vi "UI_page111.vi"(10 "传递队列输入":refnum<queue>, 11 "notifier":refnum<notifier>) -> ()   [LabVIEW 2012]
uses:
  <vilib>/GPower/VIRegister/Library/Convert/ToSGLArry.vi
  <vilib>/GPower/VIRegister/Library/Convert/ToU32.vi
  <vilib>/GPower/VIRegister/Library/SubVIs/FindRegisterData.vi
  <vilib>/GPower/VIRegister/Library/SubVIs/ReadSub.vi
  <vilib>/GPower/VIRegister/Library/SubVIs/WriteSub.vi
  <vilib>/GPower/VIRegister/Library/QManager/GetRegisterData.vi
  <vilib>/GPower/Error/Library/SetError.vi
  <vilib>/GPower/Error/Library/FilterCodes.vi
  <vilib>/GPower/Error/Library/Filter/FilterMulti.vi
  <vilib>/GPower/VIRegister/Library/QManager/QManagerAction.vi
  <vilib>/GPower/Error/Library/ErrorType.vi
  <vilib>/GPower/Error/Library/SplitAppended.vi
  <vilib>/GPower/Error/Library/SubVIs/ExplanationToError.vi
  <vilib>/GPower/VIRegister/Library/QManager/GetQName.vi
  <vilib>/GPower/VIRegister/Library/QManager/StartQManager.vi
  <vilib>/Utility/error.llb/Trim Whitespace.vi
  <vilib>/dlg_ctls.llb/Space Constant.vi
  <vilib>/Utility/error.llb/Error Code Database.vi
  <vilib>/GPower/Error/Library/SubVIs/SetStatus.vi
  <vilib>/GPower/Error/Library/AppendErrors.vi
  <vilib>/GPower/Error/Library/Append/AppendSingle.vi
  <vilib>/GPower/VIRegister/VIRegister.lvlib
panel:
  in  "备份发送上一指令字":bool
  in  "备份启动自测试":bool
  in  "备份发送自检测试字":bool
  out "备份温控健康状态":bool caption="健康状态"
  out "备份温控工作状态":bool caption="工作状态"
  out "主份温控健康状态":bool caption="健康状态"
  out "主份温控工作状态":bool caption="工作状态"
  in  "主份发送自检测试字":bool
  in  "主份启动自测试":bool
  in  "主份发送上一指令字":bool
  in  "备份地检":bool
  in  "备份1553B":bool=TRUE
  out "备份A3加电状态":bool caption="加电状态"
  out "备份A2加电状态":bool caption="加电状态"
  out "备份A1加电状态":bool caption="加电状态"
  out "备份G3加电状态":bool caption="加电状态"
  out "备份G2加电状态":bool caption="加电状态"
  out "备份G1加电状态":bool caption="加电状态"
  in  "地检":bool
  in  "1553B":bool=TRUE
  out "主份A3加电状态":bool caption="加电状态"
  out "主份A2加电状态":bool caption="加电状态"
  out "主份A1加电状态":bool caption="加电状态"
  out "主份G3加电状态":bool caption="加电状态"
  out "主份G2加电状态":bool caption="加电状态"
  out "主份G1加电状态":bool caption="加电状态"
  in  "主份复位":enum32{"On", "Off"}(radio)=enum."Off" caption="复位"
  in  "备份复位":enum32{"On", "Off"}(radio)=enum."Off" caption="复位"
  in  "备份发送控制字":bool
  in  "主份发送控制字":bool
  in  "备份加计3":enum32{"On", "Off", "Keep"}(radio)=enum."Keep" caption="加计3"
  in  "备份加计2":enum32{"On", "Off", "Keep"}(radio)=enum."Keep" caption="加计2"
  in  "备份加计1":enum32{"On", "Off", "Keep"}(radio)=enum."Keep" caption="加计1"
  in  "备份陀螺3":enum32{"On", "Off", "Keep"}(radio)=enum."Keep" caption="陀螺3"
  in  "备份陀螺2":enum32{"On", "Off", "Keep"}(radio)=enum."Keep" caption="陀螺2"
  in  "备份陀螺1":enum32{"On", "Off", "Keep"}(radio)=enum."Keep" caption="陀螺1"
  in  "备份温控":enum32{"On", "Off", "Keep"}(radio)=enum."Keep" caption="温控"
  in  "加计3":enum32{"On", "Off", "Keep"}(radio)=enum."Keep"
  in  "加计2":enum32{"On", "Off", "Keep"}(radio)=enum."Keep"
  in  "加计1":enum32{"On", "Off", "Keep"}(radio)=enum."Keep"
  in  "陀螺3":enum32{"On", "Off", "Keep"}(radio)=enum."Keep"
  in  "陀螺2":enum32{"On", "Off", "Keep"}(radio)=enum."Keep"
  in  "陀螺1":enum32{"On", "Off", "Keep"}(radio)=enum."Keep"
  in  "温控":enum32{"On", "Off", "Keep"}(radio)=enum."Keep"
  in  "备份切小量程IF电路":bool
  in  "备份切大量程IF电路":bool
  out "模拟量显示区":string
  out "备份自检状态及船舱标志":string
  out "主份自检状态及船舱标志":string
  out "接收数据统计区域":string
  in  "备份复位远程终端":bool
  in  "备份取消发送器关闭":bool
  in  "备份发送器关闭":bool
  in  "备份发送上一状态字":bool
  in  "主份复位远程终端":bool
  in  "主份取消发送器关闭":bool
  in  "主份发送器关闭":bool
  in  "主份发送上一状态字":bool
  in  "备份RT地址选择":enum32{"RT31", "RT21", "RT9"}(radio)
  in  "主份RT地址选择":enum32{"RT31", "RT21", "RT9"}(radio)
  in  "备份通道选择":enum32{"通道A", "通道B"}(radio)
  in  "主份通道选择":enum32{"通道A", "通道B"}(radio)
  in  "备份自定义周期":u16=10 caption="ms" min=10 max=480
  in  "备份周期设置":enum32{"160ms", "自定义", "480ms"}(radio)
  in  "主份自定义周期":u16=10 caption="ms" min=10 max=480
  in  "主份周期设置":enum32{"160ms", "自定义", "480ms"}(radio)
  # "主份模式指令"
  # "备份模式指令"
  # "主份指令"
  # "备份指令"
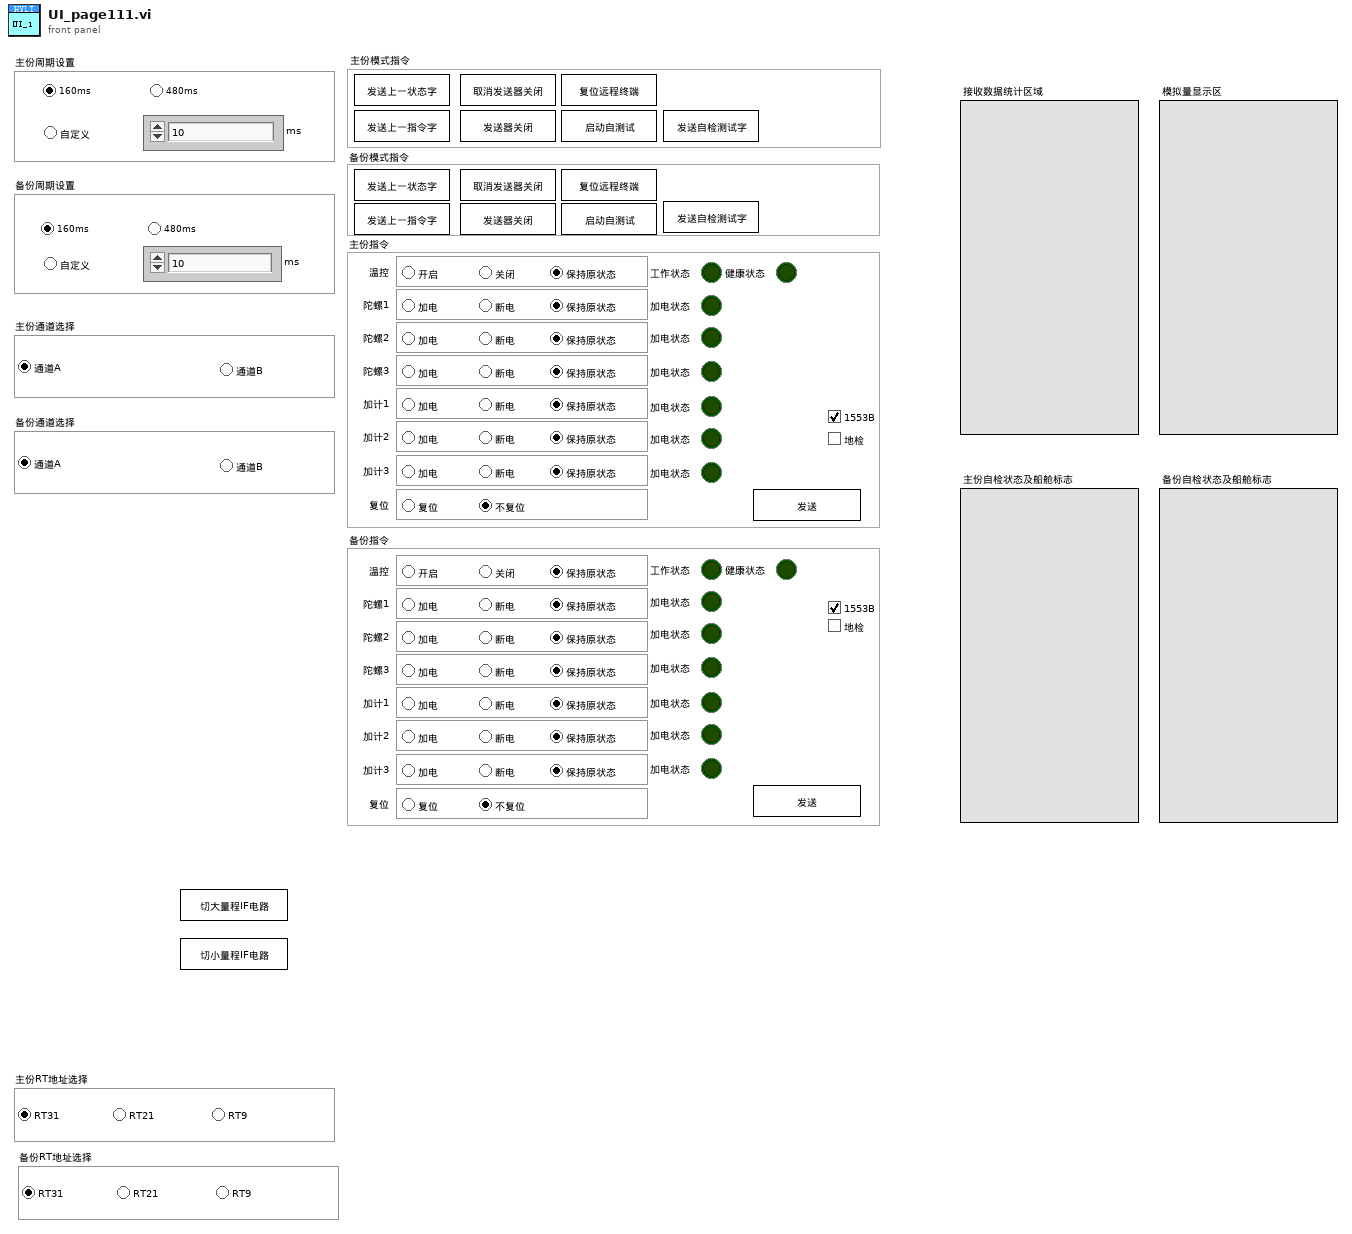
[diagram p1: front panel]
types:
  T1 = cluster{"主份通道选择":enum32{"通道A", "通道B"}, "备份通道选择":enum32{"通道A", "通道B"}}
  T2 = enum32{"invalid app kind", "Development System", "Run Time System", "Student Edition", "Embedded LabVIEW", "Evaluation", "Custom"}
  T3 = enum32{"Invalid", "Standard", "Closed", "Hidden", "Minimized", "Maximized"}
  T4 = cluster{"Core":cluster{"Current VI Reference":refnum<vi>, "Close Panel on Exit?":bool}, "传递队列输入":refnum<queue>, "信息帧":cluster{" 数据帧名称":string, " 数据":string, "备用操作符":bool, "起始地址":i32, "读写标志":i32, "长度":i32}, "主份控制指令":u16, "备份控制指令":u16, "notifier ":refnum<notifier>, "秒计数":i64, "起始时间":i64, "定时控制":bool}
  T5 = cluster{" 数据帧名称":string, " 数据":string, "备用操作符":bool, "起始地址":i32, "读写标志":i32, "长度":i32}
  T6 = cluster{"Current VI Reference":refnum<vi>, "Close Panel on Exit?":bool}
  T7 = cluster{"G1陀螺脉冲数":i32, "G2陀螺脉冲数":i32, "G3陀螺脉冲数":i32, "A1加速度计脉冲数":i16, "A2加速度计脉冲数":i16, "A3加速度计脉冲数":i16, "G1陀螺自检状态":u8, "G1陀螺光路温度":i8, "G2陀螺自检状态":u8, "G2陀螺光路温度":i8, "G3陀螺自检状态":u8, "G3陀螺光路温度":i8, "A1自检状态":u8, "A1幅值":u8, "A2自检状态":u8, "A2幅值":u8, "A3自检状态":u8, "A3幅值":u8, "IF1电路温度":i8, "IF2电路温度":i8, "IF3电路温度":i8, "温控自检字":u8, "加计温度1":i16, "加计温度2":i16, "LTU状态":u8, "帧计数":u8, "G1陀螺光路温度E-2":i16, "G2陀螺光路温度E-2":i16, "G3陀螺光路温度E-2":i16, "G1陀螺电路温度E-2":i16, "G2陀螺电路温度E-2":i16, "G3陀螺电路温度E-2":i16}
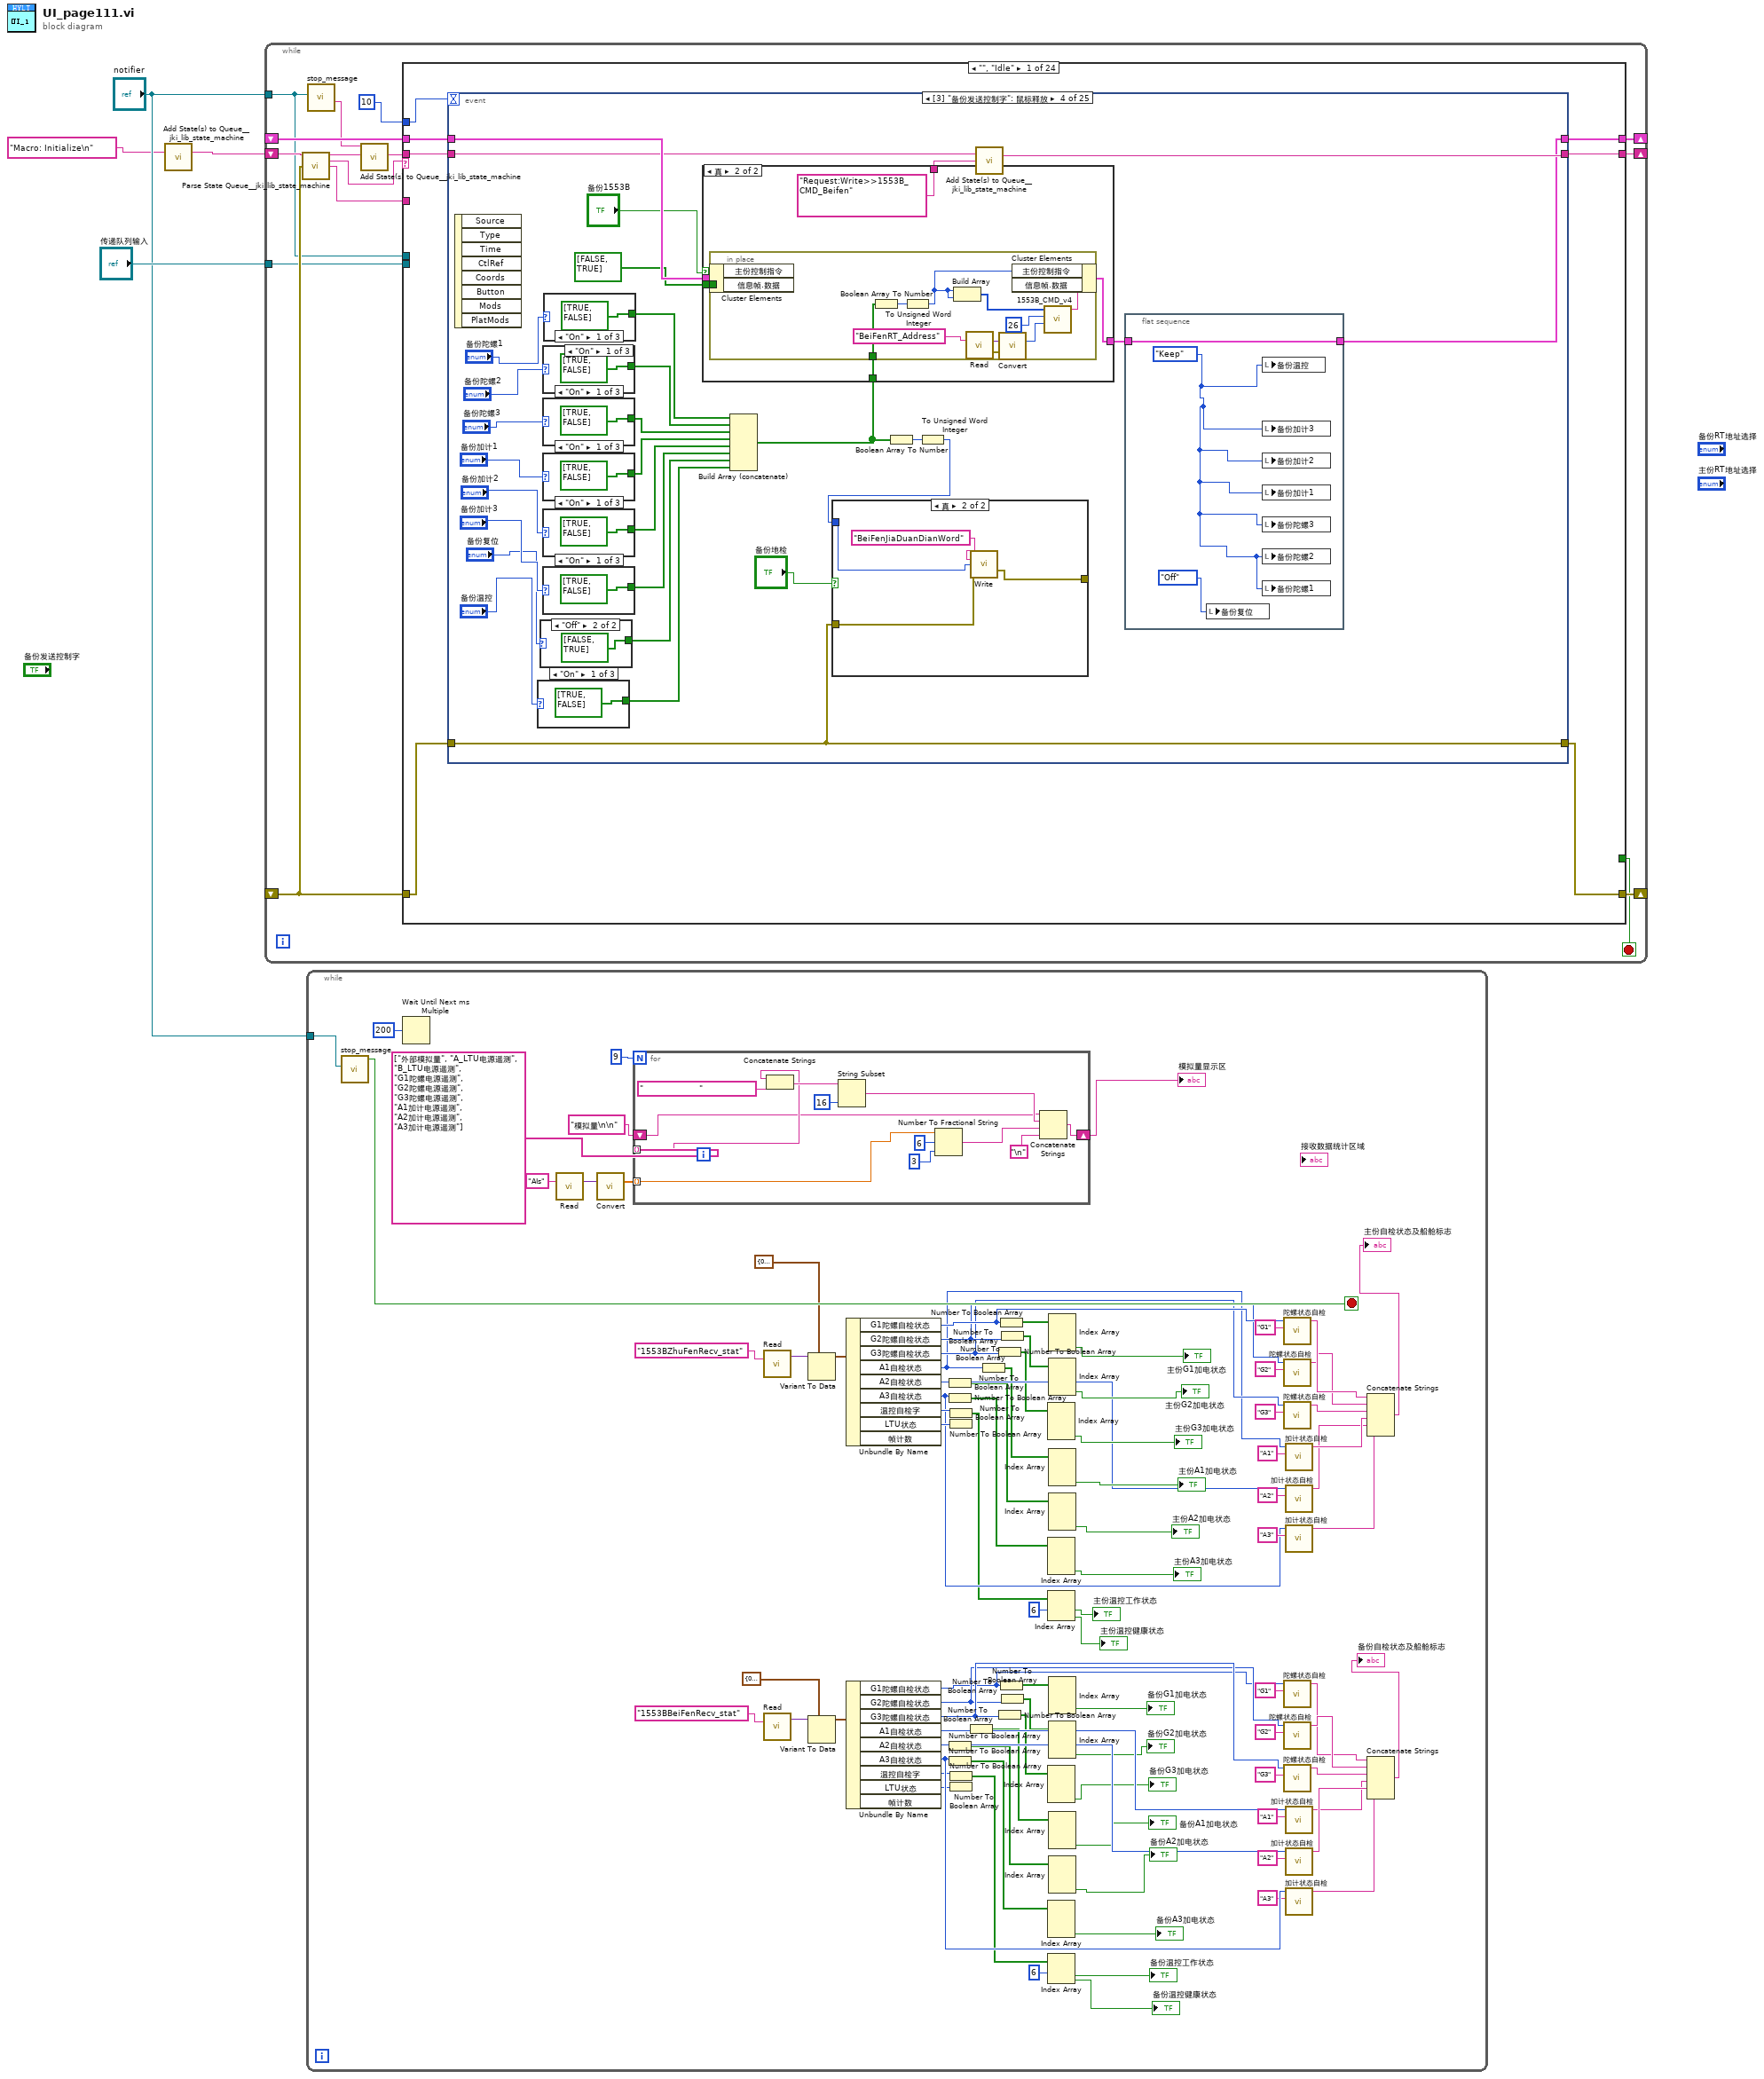
[diagram p0: block diagram]
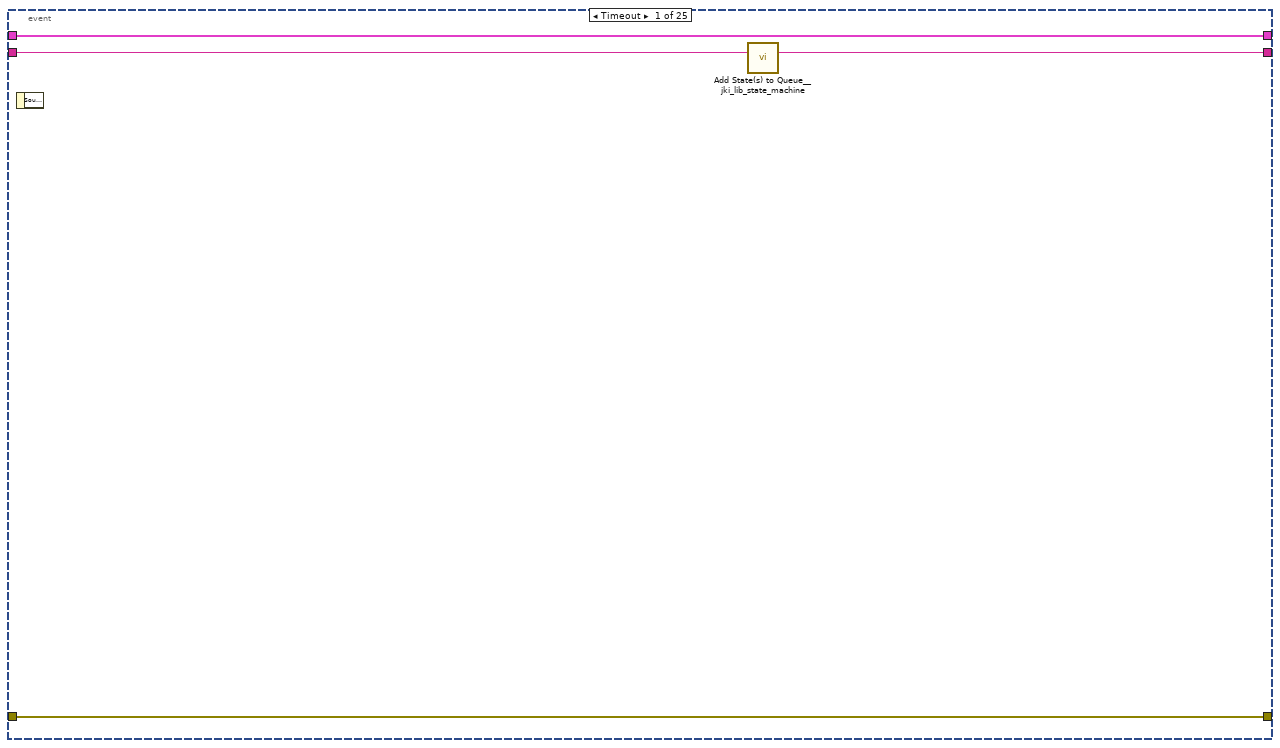
[diagram p2: hidden frame]
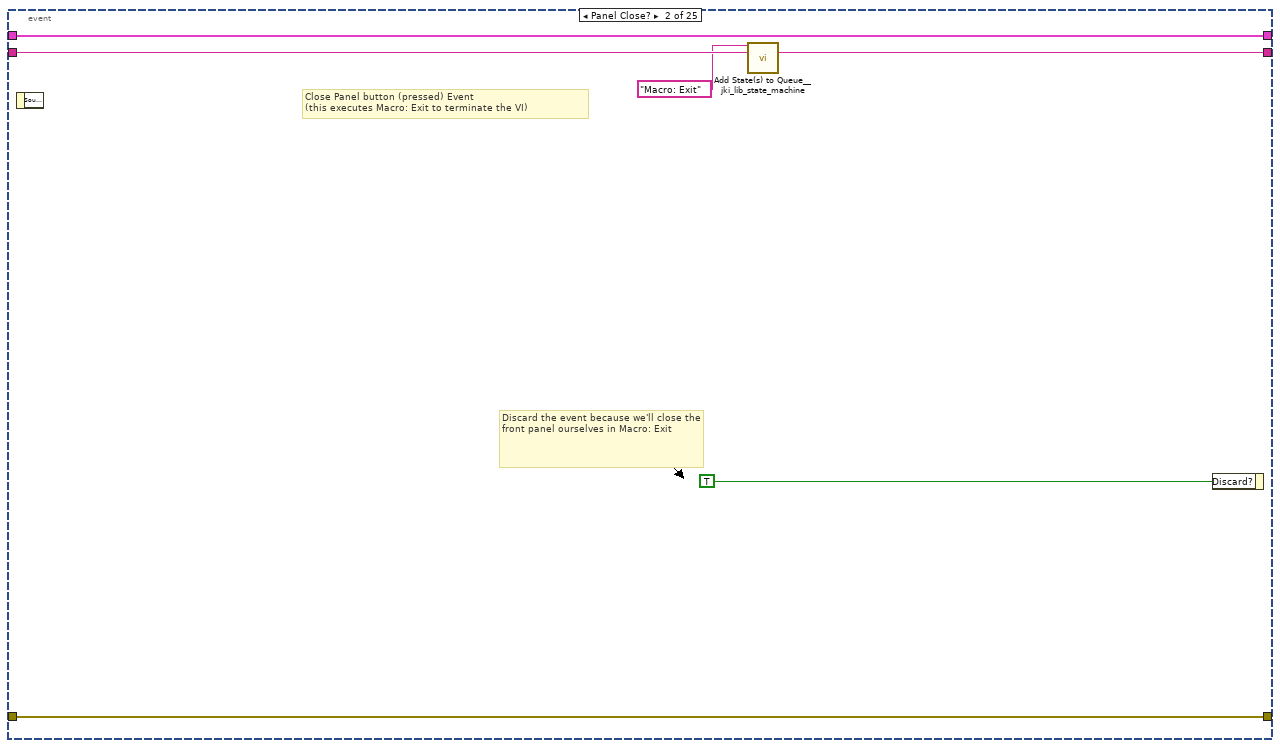
[diagram p3: hidden frame]
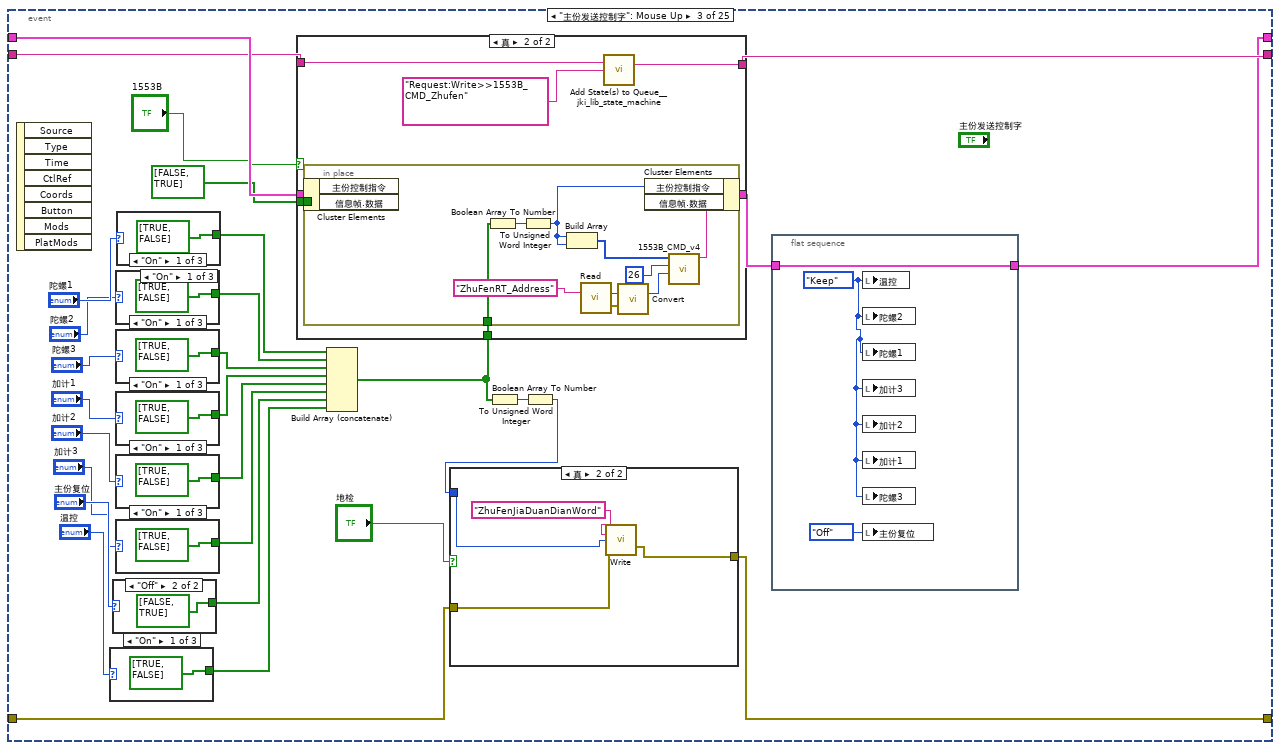
[diagram p4: hidden frame]
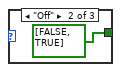
[diagram p7: hidden frame]
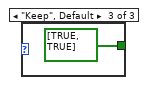
[diagram p8: hidden frame]
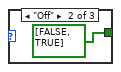
[diagram p9: hidden frame]
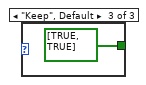
[diagram p10: hidden frame]
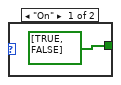
[diagram p11: hidden frame]
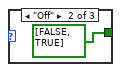
[diagram p12: hidden frame]
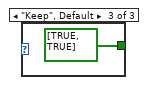
[diagram p13: hidden frame]
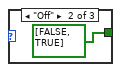
[diagram p14: hidden frame]
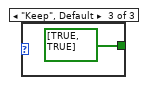
[diagram p15: hidden frame]
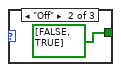
[diagram p16: hidden frame]
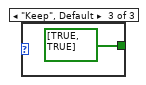
[diagram p17: hidden frame]
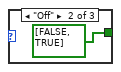
[diagram p18: hidden frame]
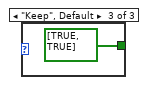
[diagram p19: hidden frame]
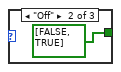
[diagram p20: hidden frame]
diagram:
  n1 = call <vilib>:"Add State(s) to Queue__jki_lib_state_machine.vi"("State(s) in (\"\")"="Macro: Initialize\n") -> ("States Out"=w4:string)  [unwired: 14 in]
  n2 = while "JKI - String-Based Queued State Machine (Basic) v1.0" {
    shift-right: [w13] -> _
    shift-left: _ -> [w12]
    shift-right: [w16] -> _
    shift-left: _ -> [w10]
    shift-right: [w15] -> _
    shift-left: w4 -> [w17]
    tunnel: "notifier" -> [w5]
    tunnel: "传递队列输入" -> [w6]
    stop <- w14 stop-if-true
    n3 = call <vilib>:"Parse State Queue__jki_lib_state_machine.vi"("State Queue"=w17, "Error In (no error)"=w10) -> ("Remaining States"=w9:string, "Current State"=w19:string, "Arguments"=w18:string)  [unwired: 11 in]
    n4 = call "stop_message.vi"("notifier"=w5) -> ("通知"=w8:string)  [unwired: 9 in, 1 out]
    n5 = call <vilib>:"Add State(s) to Queue__jki_lib_state_machine.vi"("State(s) in Front (\"\")"=w8, "State(s) in (\"\")"=w9) -> ("States Out"=w7:string)  [unwired: 13 in]
    n6 = case shown="\"\", \"Idle\"" w19 {
      selector: w19 -> [_ _ w464 _ _ _ _ _ _ _ _ _ _ _ _ _ _ _ _ _ _ _ _ _]
      tunnel: w7 -> [w20 w463 w468 w486 w492 w497 w501 w514 w520 w524 w530 w536 w546 w578 w583 w593 w597 w604 w625 w645 w664 w690 w706 w711]
      tunnel: w18 -> [_ _ _ _ _ _ _ _ _ _ _ w531 w541 _ _ _ _ w598 w619 w639 _ _ _ _]
      tunnel: w12 -> [w25 w460 w466 w477 w489 w495 w498 _ w515 w521 w528 w534 w542 w575 w580 w590 w594 w602 w623 w643 w662 w688 w703 w708]
      tunnel: [w24 w461 w470 w483 errorcluster {"status"=FALSE, "code"=0, "source"=""} ("error out") w494 w499 w511 w516 w522 w527 w532 w543 w576 w581 w591 w595 w600 w621 w641 w660 w686 w704 w709] -> w16
      tunnel: w10 -> [w23 w461 w469 w483 w488 w494 w499 w511 w517 w522 w527 w533 w544 w576 w581 w591 w595 w601 w622 w642 w661 w687 w704 w709]
      tunnel: [w26 w462 w467 w485 w491 w496 w500 w513 w519 w523 w529 w535 w545 w577 w582 w592 w596 w603 w624 w644 w663 w689 w705 w710] -> w15
      tunnel: [_ _ _ _ _ TRUE _ _ _ _ _ _ _ _ _ _ _ _ _ _ _ _ _ _] -> w14
      tunnel: [w22 w460 w466 w484 w489 w495 w498 w512 w515 w521 w528 w534 w542 w575 w580 w590 w594 w599 w620 w640 w659 w685 w703 w708] -> w13
      tunnel: 10 ("Timeout") -> [w21 _ _ _ _ _ _ _ _ _ _ _ _ _ _ _ _ _ _ _ _ _ _ _]
      tunnel: w6 -> [_ _ _ _ _ _ _ w508 _ _ _ _ _ _ _ _ _ _ _ _ _ _ _ _]
      tunnel: w5 -> [_ _ _ _ _ _ _ w505 _ _ _ _ _ _ _ _ _ _ _ _ _ _ _ _]
      frame "", "Idle" {
        n7 = event shown="[3] \"备份发送控制字\": 鼠标释放" {
          selector: _ -> [_ _ _ _ _ _ _ _ _ _ _ _ _ _ _ _ _ _ _ _ _ _ _ _ _]
          dyn-events: _ -> [_ _ _ _ _ _ _ _ _ _ _ _ _ _ _ _ _ _ _ _ _ _ _ _ _]
          timeout: w21 -> [_ _ _ _ _ _ _ _ _ _ _ _ _ _ _ _ _ _ _ _ _ _ _ _ _]
          tunnel: w20 -> [w30 w36 w64 w143 w199 w208 w215 w236 w255 w273 w284 w295 w307 w319 w331 w343 w355 w367 w379 w391 w403 w415 w427 w439 w451]
          tunnel: [w29 w35 w63 w141 w197 w206 w214 w235 w254 w272 w282 w293 w305 w317 w329 w341 w353 w365 w377 w389 w401 w413 w425 w437 w449] -> w26
          tunnel: w25 -> [w27 w33 w65 w144 w201 w210 w218 w238 w257 w270 w286 w297 w309 w321 w333 w345 w357 w369 w381 w393 w405 w417 w429 w441 w453]
          tunnel: [w28 w34 w37 w117 w196 w205 w213 w227 w246 w265 w281 w292 w304 w316 w328 w340 w352 w364 w376 w388 w400 w412 w424 w436 w448] -> w24
          tunnel: w23 -> [w28 w34 w38 w117 w196 w205 w213 w231 w249 w266 w281 w292 w304 w316 w328 w340 w352 w364 w376 w388 w400 w412 w424 w436 w448]
          tunnel: [w27 w33 w44 w130 w200 w209 w216 w237 w256 w269 w285 w296 w308 w320 w332 w344 w356 w368 w380 w392 w404 w416 w428 w440 w452] -> w22
          event Timeout {
            n8 = event-data() -> ()  [unwired: 1 in, 1 out]
            n9 = call <vilib>:"Add State(s) to Queue__jki_lib_state_machine.vi"("State(s) in (\"\")"=w30) -> ("States Out"=w29:string)  [unwired: 14 in]
          }
          event Panel Close? {
            # "Discard the event because we'll close the front panel ourselves in Macro: Exit"
            # "Close Panel button (pressed) Event\n(this executes Macro: Exit to terminate the VI)"
            n10 = event-data() -> ()  [unwired: 1 in, 1 out]
            n11 = call <vilib>:"Add State(s) to Queue__jki_lib_state_machine.vi"("State(s) in Front (\"\")"="Macro: Exit", "State(s) in (\"\")"=w36) -> ("States Out"=w35:string)  [unwired: 13 in]
            n12 = event-data("Discard?"=TRUE) -> ()  [unwired: 1 in, 1 out]
          }
          event "主份发送控制字": Mouse Up {
            n13 = event-data() -> ()  [unwired: 1 in, 8 out]
            n14 = case shown="\"On\"" "温控" {
              tunnel: [bool[] [TRUE, FALSE] bool[] [FALSE, TRUE] bool[] [TRUE, TRUE]] -> w46
              frame "On" {
              }
              frame "Off" {
              }
              frame "Keep", Default {
              }
            }
            n15 = case shown="\"Off\"" "主份复位" {
              tunnel: [bool[] [TRUE, FALSE] bool[] [FALSE, TRUE]] -> w47
              frame "On" {
              }
              frame "Off" {
              }
            }
            n16 = case shown="\"On\"" "陀螺2" {
              tunnel: [bool[] [TRUE, FALSE] bool[] [FALSE, TRUE] bool[] [TRUE, TRUE]] -> w52
              frame "On" {
              }
              frame "Off" {
              }
              frame "Keep", Default {
              }
            }
            n17 = case shown="\"On\"" "陀螺3" {
              tunnel: [bool[] [TRUE, FALSE] bool[] [FALSE, TRUE] bool[] [TRUE, TRUE]] -> w51
              frame "On" {
              }
              frame "Off" {
              }
              frame "Keep", Default {
              }
            }
            n18 = case shown="\"On\"" "加计1" {
              tunnel: [bool[] [TRUE, FALSE] bool[] [FALSE, TRUE] bool[] [TRUE, TRUE]] -> w50
              frame "On" {
              }
              frame "Off" {
              }
              frame "Keep", Default {
              }
            }
            n19 = case shown="\"On\"" "加计2" {
              tunnel: [bool[] [TRUE, FALSE] bool[] [FALSE, TRUE] bool[] [TRUE, TRUE]] -> w49
              frame "On" {
              }
              frame "Off" {
              }
              frame "Keep", Default {
              }
            }
            n20 = case shown="\"On\"" "加计3" {
              tunnel: [bool[] [TRUE, FALSE] bool[] [FALSE, TRUE] bool[] [TRUE, TRUE]] -> w48
              frame "On" {
              }
              frame "Off" {
              }
              frame "Keep", Default {
              }
            }
            n21 = case shown="\"On\"" "陀螺1" {
              tunnel: [bool[] [TRUE, FALSE] bool[] [FALSE, TRUE] bool[] [TRUE, TRUE]] -> w53
              frame "On" {
              }
              frame "Off" {
              }
              frame "Keep", Default {
              }
            }
            n22 = Build Array (concatenate)(w53, w52, w51, w50, w49, w48, w47, w46) -> (w41:bool[])
            n23 = case shown="真" "1553B" {
              tunnel: w65 -> [w71 w79]
              tunnel: w64 -> [w72 w78]
              tunnel: [w72 w76] -> w63
              tunnel: bool[] [FALSE, TRUE] -> [_ w75]
              tunnel: w41 -> [_ w74]
              tunnel: [w71 w73] -> w45
              frame False {
              }
              frame True {
                n24 = in-place {
                  in-place-border: w75 -> [_]
                  in-place-border: w74 -> [w88]
                  n25 = in-place-cluster #1(w79) -> ()  [unwired: 2 out]
                  n26 = Boolean Array To Number(Boolean array=w88) -> (number=w89:u32)
                  n27 = To Unsigned Word Integer(number=w89) -> (unsigned 16bit integer=w80:u16)
                  n28 = Build Array(w80, w80) -> (w86:u16[])
                  n29 = call <vilib>:"Read.vi"("Register name"="ZhuFenRT_Address") -> ("Register value"=w84:variant, "Error out"=w81:errorcluster)  [unwired: 11 in, 2 out]
                  n30 = call-poly <vilib>:"Convert.vi"("Register value in"=w84, "Error in"=w81) -> ("Register value out"=w83:u32)  [unwired: 12 in, 1 out]
                  n31 = call "1553B_CMD_v4.vi"("RT地址"=w83, "控制指令子地址(默认：11010"=u16 26, "数据字数组"=w86) -> ("1553B指令"=w82:string)  [unwired: 8 in]
                  n32 = in-place-cluster #1("主份控制指令"=w80, "信息帧.数据"=w82) -> (w73:T4)
                }
                n33 = call <vilib>:"Add State(s) to Queue__jki_lib_state_machine.vi"("State(s) in (\"\")"=w78, "State(s) at Back (\"\")"="Request:Write>>1553B_CMD_Zhufen") -> ("States Out"=w76:string)  [unwired: 13 in]
              }
            }
            n34 = Boolean Array To Number(Boolean array=w41) -> (number=w42:u32)
            n35 = To Unsigned Word Integer(number=w42) -> (unsigned 16bit integer=w39:u16)
            n36 = case shown="真" "地检" {
              tunnel: w39 -> [_ w69]
              tunnel: w38 -> [w66 w68]
              tunnel: [w66 w67] -> w37
              frame False {
              }
              frame True {
                n37 = call <vilib>:"Write.vi"("Register name"="ZhuFenJiaDuanDianWord", "Register value"=w69, "Error in"=w68) -> ("Error out"=w67:errorcluster)  [unwired: 10 in, 2 out]
              }
            }
            n38 = flat-sequence {
              tunnel: w45 -> [w90]
              tunnel: [w90] -> w44
              frame #0 {
                w92 = enum32{"On", "Off", "Keep"}."Keep" ("温控")
                n39 = local write "温控"(w92) -> ()
                n40 = local write "陀螺2"(w92) -> ()
                n41 = local write "陀螺1"(w92) -> ()
                n42 = local write "加计3"(w92) -> ()
                n43 = local write "加计2"(w92) -> ()
                n44 = local write "加计1"(w92) -> ()
                n45 = local write "陀螺3"(w92) -> ()
                n46 = local write "主份复位"(enum32{"On", "Off"}."Off" ("主份复位")) -> ()
              }
            }
          }
          event "备份发送控制字": Mouse Up {
            n47 = event-data() -> ()  [unwired: 1 in, 8 out]
            n48 = case shown="\"On\"" "备份温控" {
              tunnel: [bool[] [TRUE, FALSE] bool[] [FALSE, TRUE] bool[] [TRUE, TRUE]] -> w132
              frame "On" {
              }
              frame "Off" {
              }
              frame "Keep", Default {
              }
            }
            n49 = case shown="\"Off\"" "备份复位" {
              tunnel: [bool[] [TRUE, FALSE] bool[] [FALSE, TRUE]] -> w133
              frame "On" {
              }
              frame "Off" {
              }
            }
            n50 = case shown="\"On\"" "备份陀螺2" {
              tunnel: [bool[] [TRUE, FALSE] bool[] [FALSE, TRUE] bool[] [TRUE, TRUE]] -> w138
              frame "On" {
              }
              frame "Off" {
              }
              frame "Keep", Default {
              }
            }
            n51 = case shown="\"On\"" "备份陀螺3" {
              tunnel: [bool[] [TRUE, FALSE] bool[] [FALSE, TRUE] bool[] [TRUE, TRUE]] -> w137
              frame "On" {
              }
              frame "Off" {
              }
              frame "Keep", Default {
              }
            }
            n52 = case shown="\"On\"" "备份加计1" {
              tunnel: [bool[] [TRUE, FALSE] bool[] [FALSE, TRUE] bool[] [TRUE, TRUE]] -> w136
              frame "On" {
              }
              frame "Off" {
              }
              frame "Keep", Default {
              }
            }
            n53 = case shown="\"On\"" "备份加计2" {
              tunnel: [bool[] [TRUE, FALSE] bool[] [FALSE, TRUE] bool[] [TRUE, TRUE]] -> w135
              frame "On" {
              }
              frame "Off" {
              }
              frame "Keep", Default {
              }
            }
            n54 = case shown="\"On\"" "备份加计3" {
              tunnel: [bool[] [TRUE, FALSE] bool[] [FALSE, TRUE] bool[] [TRUE, TRUE]] -> w134
              frame "On" {
              }
              frame "Off" {
              }
              frame "Keep", Default {
              }
            }
            n55 = case shown="\"On\"" "备份陀螺1" {
              tunnel: [bool[] [TRUE, FALSE] bool[] [FALSE, TRUE] bool[] [TRUE, TRUE]] -> w139
              frame "On" {
              }
              frame "Off" {
              }
              frame "Keep", Default {
              }
            }
            n56 = Build Array (concatenate)(w139, w138, w137, w136, w135, w134, w133, w132) -> (w119:bool[])
            n57 = case shown="真" "备份1553B" {
              tunnel: w144 -> [w145 w151]
              tunnel: ["" "Request:Write>>1553B_CMD_Beifen"] -> w142
              tunnel: bool[] [FALSE, TRUE] -> [_ w149]
              tunnel: [w145 w148] -> w131
              tunnel: w119 -> [_ w147]
              frame False {
              }
              frame True {
                n58 = in-place {
                  in-place-border: w149 -> [_]
                  in-place-border: w147 -> [w160]
                  n59 = in-place-cluster #2(w151) -> ()  [unwired: 2 out]
                  n60 = Boolean Array To Number(Boolean array=w160) -> (number=w161:u32)
                  n61 = To Unsigned Word Integer(number=w161) -> (unsigned 16bit integer=w152:u16)
                  n62 = Build Array(w152, w152) -> (w158:u16[])
                  n63 = call <vilib>:"Read.vi"("Register name"="BeiFenRT_Address") -> ("Register value"=w157:variant, "Error out"=w155:errorcluster)  [unwired: 11 in, 2 out]
                  n64 = call-poly <vilib>:"Convert.vi"("Register value in"=w157, "Error in"=w155) -> ("Register value out"=w156:u32)  [unwired: 12 in, 1 out]
                  n65 = call "1553B_CMD_v4.vi"("RT地址"=w156, "控制指令子地址(默认：11010"=u16 26, "数据字数组"=w158) -> ("1553B指令"=w153:string)  [unwired: 8 in]
                  n66 = in-place-cluster #2("主份控制指令"=w152, "信息帧.数据"=w153) -> (w148:T4)
                }
              }
            }
            n67 = Boolean Array To Number(Boolean array=w119) -> (number=w120:u32)
            n68 = To Unsigned Word Integer(number=w120) -> (unsigned 16bit integer=w118:u16)
            n69 = case shown="真" "备份地检" {
              tunnel: w118 -> [_ w165]
              tunnel: w117 -> [w162 w164]
              tunnel: [w162 w163] -> _
              frame False {
              }
              frame True {
                n70 = call <vilib>:"Write.vi"("Register name"="BeiFenJiaDuanDianWord", "Register value"=w165, "Error in"=w164) -> ("Error out"=w163:errorcluster)  [unwired: 10 in, 2 out]
              }
            }
            n71 = call <vilib>:"Add State(s) to Queue__jki_lib_state_machine.vi"("State(s) in (\"\")"=w143, "State(s) at Back (\"\")"=w142) -> ("States Out"=w141:string)  [unwired: 13 in]
            n72 = flat-sequence {
              tunnel: w131 -> [w169]
              tunnel: [w169] -> w130
              frame #0 {
                w167 = enum32{"On", "Off", "Keep"}."Keep" ("温控")
                n73 = local write "备份复位"(enum32{"On", "Off"}."Off" ("主份复位")) -> ()
                n74 = local write "备份温控"(w167) -> ()
                n75 = local write "备份加计3"(w167) -> ()
                n76 = local write "备份加计2"(w167) -> ()
                n77 = local write "备份加计1"(w167) -> ()
                n78 = local write "备份陀螺3"(w167) -> ()
                n79 = local write "备份陀螺2"(w167) -> ()
                n80 = local write "备份陀螺1"(w167) -> ()
              }
            }
          }
          event "备份切大量程IF电路": Value Change {
            n81 = event-data() -> ()  [unwired: 1 in, 6 out]
            n82 = call "1553B_CMD_v4.vi"("控制指令子地址(默认：11010"=u16 26, "数据字数组"=u16[] [45489]) -> ("1553B指令"=w193:string)  [unwired: 9 in]
            n83 = call <vilib>:"Add State(s) to Queue__jki_lib_state_machine.vi"("State(s) in (\"\")"=w199, "State(s) at Back (\"\")"="Request:Write>>1553B_CMD_Beifen") -> ("States Out"=w197:string)  [unwired: 13 in]
            n84 = Bundle By Name(cluster=w201, "信息帧.数据"=w193) -> (w200:T4)
          }
          event "备份切小量程IF电路": Value Change {
            n85 = event-data() -> ()  [unwired: 1 in, 6 out]
            n86 = call "1553B_CMD_v4.vi"("控制指令子地址(默认：11010"=u16 26, "数据字数组"=u16[] [47802]) -> ("1553B指令"=w202:string)  [unwired: 9 in]
            n87 = call <vilib>:"Add State(s) to Queue__jki_lib_state_machine.vi"("State(s) in (\"\")"=w208, "State(s) at Back (\"\")"="Request:Write>>1553B_CMD_Beifen") -> ("States Out"=w206:string)  [unwired: 13 in]
            n88 = Bundle By Name(cluster=w210, "信息帧.数据"=w202) -> (w209:T4)
          }
          event "主份自定义周期": Value Change {
            n89 = event-data() -> ("NewVal"=w217:u16)  [unwired: 1 in, 5 out]
            n90 = property on="主份周期设置" class="RadioBtnsControl (严格)"() -> ("Value"=w212:enum32{"160ms", "自定义", "480ms"})  [unwired: 2 in, 2 out]
            n91 = case shown="\"自定义\"" w212 {
              tunnel: w218 -> [w220 w226]
              tunnel: w217 -> [_ w221]
              tunnel: [w220 w225] -> w216
              tunnel: ["" "Config:Write>>1553B_CMD_Zhufen"] -> w211
              frame "160ms", Default {
              }
              frame "自定义" {
                n92 = Number To Decimal String(number=w221) -> (decimal integer string=w224:string)  [unwired: 1 in]
                n93 = Bundle By Name(cluster=w226, "信息帧.数据"=w224) -> (w225:T4)
                n94 = call <vilib>:"Write.vi"("Register name"="Zhufen_period", "Register value"=w221) -> ()  [unwired: 11 in, 3 out]
              }
            }
            n95 = call <vilib>:"Add State(s) to Queue__jki_lib_state_machine.vi"("State(s) in (\"\")"=w215, "State(s) at Back (\"\")"=w211) -> ("States Out"=w214:string)  [unwired: 13 in]
          }
          event "主份周期设置": Value Change {
            n96 = event-data() -> ("NewVal"=w233:enum32{"160ms", "自定义", "480ms"})  [unwired: 1 in, 5 out]
            n97 = case shown="\"自定义\"" w233 {
              tunnel: [u16 160 ("Value") u16 480 ("Value") w245] -> w229
              tunnel: w231 -> [w239 w241 w244]
              tunnel: [w239 w241 w243] -> w228
              frame "160ms", Default {
              }
              frame "480ms" {
              }
              frame "自定义" {
                n98 = property on="主份自定义周期" class="DigNum (严格)"(error in=w244) -> (error out=w243:errorcluster, "Value"=w245:u16)  [unwired: 1 in, 1 out]
              }
            }
            n99 = Number To Decimal String(number=w229) -> (decimal integer string=w232:string)  [unwired: 1 in]
            n100 = Bundle By Name(cluster=w238, "信息帧.数据"=w232) -> (w237:T4)
            n101 = call <vilib>:"Add State(s) to Queue__jki_lib_state_machine.vi"("State(s) in (\"\")"=w236, "State(s) at Back (\"\")"="Config:Write>>1553B_CMD_Zhufen") -> ("States Out"=w235:string)  [unwired: 13 in]
            n102 = call <vilib>:"Write.vi"("Register name"="Zhufen_period", "Register value"=w229, "Error in"=w228) -> ("Error out"=w227:errorcluster)  [unwired: 10 in, 2 out]
          }
          event "备份周期设置": Value Change {
            n103 = event-data() -> ("NewVal"=w248:enum32{"160ms", "自定义", "480ms"})  [unwired: 1 in, 5 out]
            n104 = case shown="\"480ms\"" w248 {
              tunnel: [u16 160 ("Value") u16 480 ("Value") w264] -> w251
              tunnel: w249 -> [w258 w260 w263]
              tunnel: [w258 w260 w262] -> w250
              frame "160ms", Default {
              }
              frame "480ms" {
              }
              frame "自定义" {
                n105 = property on="备份自定义周期" class="DigNum (严格)"(error in=w263) -> (error out=w262:errorcluster, "Value"=w264:u16)  [unwired: 1 in, 1 out]
              }
            }
            n106 = call <vilib>:"Add State(s) to Queue__jki_lib_state_machine.vi"("State(s) in (\"\")"=w255, "State(s) at Back (\"\")"="Config:Write>>1553B_CMD_Beifen") -> ("States Out"=w254:string)  [unwired: 13 in]
            n107 = Number To Decimal String(number=w251) -> (decimal integer string=w247:string)  [unwired: 1 in]
            n108 = Bundle By Name(cluster=w257, "信息帧.数据"=w247) -> (w256:T4)
            n109 = call <vilib>:"Write.vi"("Register name"="Beifen_period", "Register value"=w251, "Error in"=w250) -> ("Error out"=w246:errorcluster)  [unwired: 10 in, 2 out]
          }
          event "备份自定义周期": Value Change {
            n110 = event-data() -> ("NewVal"=w268:u16)  [unwired: 1 in, 5 out]
            n111 = property on="备份周期设置" class="RadioBtnsControl (严格)"(error in=w266) -> (error out=w265:errorcluster, "Value"=w267:enum32{"160ms", "自定义", "480ms"})  [unwired: 1 in, 1 out]
            n112 = case shown="\"自定义\"" w267 {
              tunnel: w270 -> [w275 w280]
              tunnel: w268 -> [_ w279]
              tunnel: [w275 w278] -> w269
              tunnel: ["" "Config:Write>>1553B_CMD_Beifen"] -> w271
              frame "160ms", Default {
              }
              frame "自定义" {
                n113 = Number To Decimal String(number=w279) -> (decimal integer string=w277:string)  [unwired: 1 in]
                n114 = Bundle By Name(cluster=w280, "信息帧.数据"=w277) -> (w278:T4)
              }
            }
            n115 = call <vilib>:"Add State(s) to Queue__jki_lib_state_machine.vi"("State(s) in (\"\")"=w273, "State(s) at Back (\"\")"=w271) -> ("States Out"=w272:string)  [unwired: 13 in]
          }
          event "主份通道选择", "备份通道选择": Value Change {
            # "Request:OPEN1553B>>1553B_CMD_Zhufen\nRequest:OPEN1553B>>1553B_CMD_Beifen"
            n116 = event-data() -> ()  [unwired: 1 in, 6 out]
            n117 = in-place {
              n118 = in-place-cluster #3(w286) -> ()  [unwired: 1 out]
              n119 = Bundle By Name(cluster=T1 {"主份通道选择"=enum."通道A", "备份通道选择"=enum."通道B"} ("输入簇"), "主份通道选择"="主份通道选择", "备份通道选择"="备份通道选择") -> (w288:T1)
              n120 = Flatten To String(anything=w288) -> (data string=w287:string)  [unwired: 3 in, 2 out]
              n121 = in-place-cluster #3("信息帧.数据"=w287) -> (w285:T4)
            }
            n122 = call <vilib>:"Add State(s) to Queue__jki_lib_state_machine.vi"("State(s) in (\"\")"=w284, "State(s) at Back (\"\")"="Request:Write>>SwitchChanel\n") -> ("States Out"=w282:string)  [unwired: 13 in]
          }
          event "主份复位远程终端": Value Change {
            n123 = event-data() -> ()  [unwired: 1 in, 6 out]
            n124 = in-place {
              n125 = in-place-cluster #4(w297) -> ()  [unwired: 1 out]
              n126 = call <vilib>:"Read.vi"("Register name"="ZhuFenRT_Address") -> ("Register value"=w301:variant, "Error out"=w300:errorcluster)  [unwired: 11 in, 2 out]
              n127 = call-poly <vilib>:"Convert.vi"("Register value in"=w301, "Error in"=w300) -> ("Register value out"=w298:u32)  [unwired: 12 in, 1 out]
              n128 = call "1553B_Mode.vi"("模式命令"=u16 8, "RT地址"=w298) -> ("1553B指令"=w302:string)  [unwired: 9 in]
              n129 = in-place-cluster #4("信息帧.数据"=w302) -> (w296:T4)
            }
            n130 = call <vilib>:"Add State(s) to Queue__jki_lib_state_machine.vi"("State(s) in (\"\")"=w295, "State(s) at Back (\"\")"="Request:Write>>1553B_CMD_Zhufen") -> ("States Out"=w293:string)  [unwired: 13 in]
          }
          event "备份复位远程终端": Value Change {
            n131 = event-data() -> ()  [unwired: 1 in, 6 out]
            n132 = in-place {
              n133 = in-place-cluster #5(w309) -> ()  [unwired: 1 out]
              n134 = call <vilib>:"Read.vi"("Register name"="BeiFenRT_Address") -> ("Register value"=w314:variant, "Error out"=w313:errorcluster)  [unwired: 11 in, 2 out]
              n135 = call-poly <vilib>:"Convert.vi"("Register value in"=w314, "Error in"=w313) -> ("Register value out"=w312:u32)  [unwired: 12 in, 1 out]
              n136 = call "1553B_Mode.vi"("模式命令"=u16 8, "RT地址"=w312) -> ("1553B指令"=w311:string)  [unwired: 9 in]
              n137 = in-place-cluster #5("信息帧.数据"=w311) -> (w308:T4)
            }
            n138 = call <vilib>:"Add State(s) to Queue__jki_lib_state_machine.vi"("State(s) in (\"\")"=w307, "State(s) at Back (\"\")"="Request:Write>>1553B_CMD_Beifen") -> ("States Out"=w305:string)  [unwired: 13 in]
          }
          event "主份发送器关闭": Value Change {
            n139 = event-data() -> ()  [unwired: 1 in, 6 out]
            n140 = in-place {
              n141 = in-place-cluster #6(w321) -> ()  [unwired: 1 out]
              n142 = call <vilib>:"Read.vi"("Register name"="ZhuFenRT_Address") -> ("Register value"=w325:variant, "Error out"=w324:errorcluster)  [unwired: 11 in, 2 out]
              n143 = call-poly <vilib>:"Convert.vi"("Register value in"=w325, "Error in"=w324) -> ("Register value out"=w322:u32)  [unwired: 12 in, 1 out]
              n144 = call "1553B_Mode.vi"("模式命令"=u16 4, "RT地址"=w322) -> ("1553B指令"=w326:string)  [unwired: 9 in]
              n145 = in-place-cluster #6("信息帧.数据"=w326) -> (w320:T4)
            }
            n146 = call <vilib>:"Add State(s) to Queue__jki_lib_state_machine.vi"("State(s) in (\"\")"=w319, "State(s) at Back (\"\")"="Request:Write>>1553B_CMD_Zhufen") -> ("States Out"=w317:string)  [unwired: 13 in]
          }
          event "主份发送上一指令字": Value Change {
            n147 = event-data() -> ()  [unwired: 1 in, 6 out]
            n148 = in-place {
              n149 = in-place-cluster #7(w333) -> ()  [unwired: 1 out]
              n150 = call <vilib>:"Read.vi"("Register name"="ZhuFenRT_Address") -> ("Register value"=w337:variant, "Error out"=w336:errorcluster)  [unwired: 11 in, 2 out]
              n151 = call-poly <vilib>:"Convert.vi"("Register value in"=w337, "Error in"=w336) -> ("Register value out"=w334:u32)  [unwired: 12 in, 1 out]
              n152 = call "1553B_Mode.vi"("模式命令"=u16 18, "RT地址"=w334) -> ("1553B指令"=w338:string)  [unwired: 9 in]
              n153 = in-place-cluster #7("信息帧.数据"=w338) -> (w332:T4)
            }
            n154 = call <vilib>:"Add State(s) to Queue__jki_lib_state_machine.vi"("State(s) in (\"\")"=w331, "State(s) at Back (\"\")"="Request:Write>>1553B_CMD_Zhufen") -> ("States Out"=w329:string)  [unwired: 13 in]
          }
          event "备份发送上一指令字": Value Change {
            n155 = event-data() -> ()  [unwired: 1 in, 6 out]
            n156 = in-place {
              n157 = in-place-cluster #8(w345) -> ()  [unwired: 1 out]
              n158 = call <vilib>:"Read.vi"("Register name"="BeiFenRT_Address") -> ("Register value"=w349:variant, "Error out"=w348:errorcluster)  [unwired: 11 in, 2 out]
              n159 = call-poly <vilib>:"Convert.vi"("Register value in"=w349, "Error in"=w348) -> ("Register value out"=w346:u32)  [unwired: 12 in, 1 out]
              n160 = call "1553B_Mode.vi"("模式命令"=u16 18, "RT地址"=w346) -> ("1553B指令"=w350:string)  [unwired: 9 in]
              n161 = in-place-cluster #8("信息帧.数据"=w350) -> (w344:T4)
            }
            n162 = call <vilib>:"Add State(s) to Queue__jki_lib_state_machine.vi"("State(s) in (\"\")"=w343, "State(s) at Back (\"\")"="Request:Write>>1553B_CMD_Zhufen") -> ("States Out"=w341:string)  [unwired: 13 in]
          }
          event "主份启动自测试": Value Change {
            n163 = event-data() -> ()  [unwired: 1 in, 6 out]
            n164 = in-place {
              n165 = in-place-cluster #9(w357) -> ()  [unwired: 1 out]
              n166 = call <vilib>:"Read.vi"("Register name"="ZhuFenRT_Address") -> ("Register value"=w361:variant, "Error out"=w360:errorcluster)  [unwired: 11 in, 2 out]
              n167 = call-poly <vilib>:"Convert.vi"("Register value in"=w361, "Error in"=w360) -> ("Register value out"=w358:u32)  [unwired: 12 in, 1 out]
              n168 = call "1553B_Mode.vi"("模式命令"=u16 3, "RT地址"=w358) -> ("1553B指令"=w362:string)  [unwired: 9 in]
              n169 = in-place-cluster #9("信息帧.数据"=w362) -> (w356:T4)
            }
            n170 = call <vilib>:"Add State(s) to Queue__jki_lib_state_machine.vi"("State(s) in (\"\")"=w355, "State(s) at Back (\"\")"="Request:Write>>1553B_CMD_Zhufen") -> ("States Out"=w353:string)  [unwired: 13 in]
          }
          event "备份启动自测试": Value Change {
            n171 = event-data() -> ()  [unwired: 1 in, 6 out]
            n172 = in-place {
              n173 = in-place-cluster #10(w369) -> ()  [unwired: 1 out]
              n174 = call <vilib>:"Read.vi"("Register name"="BeiFenRT_Address") -> ("Register value"=w373:variant, "Error out"=w372:errorcluster)  [unwired: 11 in, 2 out]
              n175 = call-poly <vilib>:"Convert.vi"("Register value in"=w373, "Error in"=w372) -> ("Register value out"=w370:u32)  [unwired: 12 in, 1 out]
              n176 = call "1553B_Mode.vi"("模式命令"=u16 3, "RT地址"=w370) -> ("1553B指令"=w374:string)  [unwired: 9 in]
              n177 = in-place-cluster #10("信息帧.数据"=w374) -> (w368:T4)
            }
            n178 = call <vilib>:"Add State(s) to Queue__jki_lib_state_machine.vi"("State(s) in (\"\")"=w367, "State(s) at Back (\"\")"="Request:Write>>1553B_CMD_Zhufen") -> ("States Out"=w365:string)  [unwired: 13 in]
          }
          event "主份发送自检测试字": Value Change {
            n179 = event-data() -> ()  [unwired: 1 in, 6 out]
            n180 = in-place {
              n181 = in-place-cluster #11(w381) -> ()  [unwired: 1 out]
              n182 = call <vilib>:"Read.vi"("Register name"="ZhuFenRT_Address") -> ("Register value"=w385:variant, "Error out"=w384:errorcluster)  [unwired: 11 in, 2 out]
              n183 = call-poly <vilib>:"Convert.vi"("Register value in"=w385, "Error in"=w384) -> ("Register value out"=w382:u32)  [unwired: 12 in, 1 out]
              n184 = call "1553B_Mode.vi"("模式命令"=u16 11, "RT地址"=w382) -> ("1553B指令"=w386:string)  [unwired: 9 in]
              n185 = in-place-cluster #11("信息帧.数据"=w386) -> (w380:T4)
            }
            n186 = call <vilib>:"Add State(s) to Queue__jki_lib_state_machine.vi"("State(s) in (\"\")"=w379, "State(s) at Back (\"\")"="Request:Write>>1553B_CMD_Zhufen") -> ("States Out"=w377:string)  [unwired: 13 in]
          }
          event "备份发送自检测试字": Value Change {
            n187 = event-data() -> ()  [unwired: 1 in, 6 out]
            n188 = in-place {
              n189 = in-place-cluster #12(w393) -> ()  [unwired: 1 out]
              n190 = call <vilib>:"Read.vi"("Register name"="BeiFenRT_Address") -> ("Register value"=w397:variant, "Error out"=w396:errorcluster)  [unwired: 11 in, 2 out]
              n191 = call-poly <vilib>:"Convert.vi"("Register value in"=w397, "Error in"=w396) -> ("Register value out"=w394:u32)  [unwired: 12 in, 1 out]
              n192 = call "1553B_Mode.vi"("模式命令"=u16 11, "RT地址"=w394) -> ("1553B指令"=w398:string)  [unwired: 9 in]
              n193 = in-place-cluster #12("信息帧.数据"=w398) -> (w392:T4)
            }
            n194 = call <vilib>:"Add State(s) to Queue__jki_lib_state_machine.vi"("State(s) in (\"\")"=w391, "State(s) at Back (\"\")"="Request:Write>>1553B_CMD_Zhufen") -> ("States Out"=w389:string)  [unwired: 13 in]
          }
          event "备份发送器关闭": Value Change {
            n195 = event-data() -> ()  [unwired: 1 in, 6 out]
            n196 = in-place {
              n197 = in-place-cluster #13(w405) -> ()  [unwired: 1 out]
              n198 = call <vilib>:"Read.vi"("Register name"="BeiFenRT_Address") -> ("Register value"=w409:variant, "Error out"=w408:errorcluster)  [unwired: 11 in, 2 out]
              n199 = call-poly <vilib>:"Convert.vi"("Register value in"=w409, "Error in"=w408) -> ("Register value out"=w406:u32)  [unwired: 12 in, 1 out]
              n200 = call "1553B_Mode.vi"("模式命令"=u16 4, "RT地址"=w406) -> ("1553B指令"=w410:string)  [unwired: 9 in]
              n201 = in-place-cluster #13("信息帧.数据"=w410) -> (w404:T4)
            }
            n202 = call <vilib>:"Add State(s) to Queue__jki_lib_state_machine.vi"("State(s) in (\"\")"=w403, "State(s) at Back (\"\")"="Request:Write>>1553B_CMD_Beifen") -> ("States Out"=w401:string)  [unwired: 13 in]
          }
          event "主份取消发送器关闭": Value Change {
            n203 = event-data() -> ()  [unwired: 1 in, 6 out]
            n204 = in-place {
              n205 = in-place-cluster #14(w417) -> ()  [unwired: 1 out]
              n206 = call <vilib>:"Read.vi"("Register name"="ZhuFenRT_Address") -> ("Register value"=w421:variant, "Error out"=w420:errorcluster)  [unwired: 11 in, 2 out]
              n207 = call-poly <vilib>:"Convert.vi"("Register value in"=w421, "Error in"=w420) -> ("Register value out"=w418:u32)  [unwired: 12 in, 1 out]
              n208 = call "1553B_Mode.vi"("模式命令"=u16 5, "RT地址"=w418) -> ("1553B指令"=w422:string)  [unwired: 9 in]
              n209 = in-place-cluster #14("信息帧.数据"=w422) -> (w416:T4)
            }
            n210 = call <vilib>:"Add State(s) to Queue__jki_lib_state_machine.vi"("State(s) in (\"\")"=w415, "State(s) at Back (\"\")"="Request:Write>>1553B_CMD_Zhufen") -> ("States Out"=w413:string)  [unwired: 13 in]
          }
          event "备份取消发送器关闭": Value Change {
            n211 = event-data() -> ()  [unwired: 1 in, 6 out]
            n212 = in-place {
              n213 = in-place-cluster #15(w429) -> ()  [unwired: 1 out]
              n214 = call <vilib>:"Read.vi"("Register name"="BeiFenRT_Address") -> ("Register value"=w433:variant, "Error out"=w432:errorcluster)  [unwired: 11 in, 2 out]
              n215 = call-poly <vilib>:"Convert.vi"("Register value in"=w433, "Error in"=w432) -> ("Register value out"=w430:u32)  [unwired: 12 in, 1 out]
              n216 = call "1553B_Mode.vi"("模式命令"=u16 5, "RT地址"=w430) -> ("1553B指令"=w434:string)  [unwired: 9 in]
              n217 = in-place-cluster #15("信息帧.数据"=w434) -> (w428:T4)
            }
            n218 = call <vilib>:"Add State(s) to Queue__jki_lib_state_machine.vi"("State(s) in (\"\")"=w427, "State(s) at Back (\"\")"="Request:Write>>1553B_CMD_Beifen") -> ("States Out"=w425:string)  [unwired: 13 in]
          }
          event "主份发送上一状态字": Value Change {
            n219 = event-data() -> ()  [unwired: 1 in, 6 out]
            n220 = in-place {
              n221 = in-place-cluster #16(w441) -> ()  [unwired: 1 out]
              n222 = call <vilib>:"Read.vi"("Register name"="ZhuFenRT_Address") -> ("Register value"=w445:variant, "Error out"=w444:errorcluster)  [unwired: 11 in, 2 out]
              n223 = call-poly <vilib>:"Convert.vi"("Register value in"=w445, "Error in"=w444) -> ("Register value out"=w442:u32)  [unwired: 12 in, 1 out]
              n224 = call "1553B_Mode.vi"("模式命令"=u16 2, "RT地址"=w442) -> ("1553B指令"=w446:string)  [unwired: 9 in]
              n225 = in-place-cluster #16("信息帧.数据"=w446) -> (w440:T4)
            }
            n226 = call <vilib>:"Add State(s) to Queue__jki_lib_state_machine.vi"("State(s) in (\"\")"=w439, "State(s) at Back (\"\")"="Request:Write>>1553B_CMD_Zhufen") -> ("States Out"=w437:string)  [unwired: 13 in]
          }
          event "备份发送上一状态字": Value Change {
            n227 = event-data() -> ()  [unwired: 1 in, 6 out]
            n228 = in-place {
              n229 = in-place-cluster #17(w453) -> ()  [unwired: 1 out]
              n230 = call <vilib>:"Read.vi"("Register name"="BeiFenRT_Address") -> ("Register value"=w457:variant, "Error out"=w456:errorcluster)  [unwired: 11 in, 2 out]
              n231 = call-poly <vilib>:"Convert.vi"("Register value in"=w457, "Error in"=w456) -> ("Register value out"=w454:u32)  [unwired: 12 in, 1 out]
              n232 = call "1553B_Mode.vi"("模式命令"=u16 2, "RT地址"=w454) -> ("1553B指令"=w458:string)  [unwired: 9 in]
              n233 = in-place-cluster #17("信息帧.数据"=w458) -> (w452:T4)
            }
            n234 = call <vilib>:"Add State(s) to Queue__jki_lib_state_machine.vi"("State(s) in (\"\")"=w451, "State(s) at Back (\"\")"="Request:Write>>1553B_CMD_Beifen") -> ("States Out"=w449:string)  [unwired: 13 in]
          }
        }
      }
      frame "---------- Core ----------" {
        # "Do not put any code in this frame.\n(it is a separator no-op)"
        n235 = call <vilib>:"Add State(s) to Queue__jki_lib_state_machine.vi"("State(s) in (\"\")"=w463) -> ("States Out"=w462:string)  [unwired: 14 in]
      }
      frame Default {
        w473 = 42 items=["No error", "Argument error", "Memory is full", "Out of zone", "End of file", "File already open", "Generic file I/O error", "File not found", "File permission error", "Disk is full", "Duplicate path", "Too many files open", "System feature not enabled", "Resource file not found", "Cannot add resource", "Resource not found", "Image not found", "Image memory error", "Pen does not exist", "Config type invalid", "Config token not found", "Config parse error", "Config memory error", "Bad external code format", "Bad external code offset", "External code not present", "Null window", "Destroy window error", "Null menu", "Print aborted", "Bad print record", "Print driver error", "Windows error during printing", "Memory error during printing", "Print dialog error", "Generic print error", "Invalid device refnum", "Device not found", "Device parameter error", "Device unit error", "Cannot open device", "Device call aborted", "Generic error", "Cancelled by user", "Object ID too low", "Object ID too high", "Object not in heap", "Unknown heap", "Unknown object (invalid DefProc)", "Unknown object (DefProc not in table)", "Message out of range", "Invalid (null) method", "Unknown message", "Manager call not supported", "Bad address", "Network operation in progress", "Network operation timed out", "Connection is busy", "Network attribute not supported", "Network error", "Address in use", "System out of memory", "Connection aborted", "Connection refused", "Not connected", "Already connected", "Connection closed", "Initialization error (interapplication manager)", "Bad occurrence", "Wait on unbound occurrence handler", "Occurrence queue overflow", "Datalog type conflict", "Unused", "Unrecognized type (interapplication manager)", "Memory corrupt", "Failed to make temporary DLL", "Old CIN version", "Drag socket not found", "Failed to load drop-object", "Failed to register OLE object", "Failed to release OLE object", "Format specifier type mismatch", "Unknown format specifier", "Too few format specifiers", "Too many format specifiers", "Scan failed", "Newer CIN version", "Error converting to variant", "Runtime menu error", "Password tampered", "Variant attribute not found", "Incompatible variant data type", "Event data is not available", "Event Store is not present", "Occurrence is not found", "Event Queue is not created", "Event info is not available", "Refnum passed is NULL", "Error retrieving Class GUID", "Error retrieving CoClass GUID", "Error retrieving TypeLib GUID.", "Bad built application magic bytes.", "Specific driver is different from the specific driver associated with the Logical Name.", "There is no session opened to the class driver.", "Max Error", "MAX - Error with config objects", "MAX - Error loading configuration", "MAX - Group not supported"]
        # "Current State"
        # "Do not delete, rename, or modify this frame.\n(this is used to capture unhandled states and typos)"
        # "Handle mistyped state name (developer tool)"
        n236 = Format Into String(format string="Software Exception: Unhandled State \"%s\"." ("message"), error in=w469, w464) -> (resulting string=w472:string, error out=w471:errorcluster)  [unwired: 1 in]
        n237 = call <vilib>:"Error Cluster From Error Code.vi"("show call chain? (False)"=TRUE, "error in (no error)"=w471, "error message (\"\")"=w472, "error code (0)"=w473) -> ("error out"=w470:errorcluster)  [unwired: 5 in]
        n238 = call <vilib>:"Add State(s) to Queue__jki_lib_state_machine.vi"("State(s) in (\"\")"=w468) -> ("States Out"=w467:string)  [unwired: 14 in]
      }
      frame "Initialize Core Data" {
        # "Do not delete, rename, or modify this frame.\n(this is used to determine panel behavior on exit)"
        # "originally closed?"
        # "exe?"
        # "If panel starts closed or is an EXE, then close it when we exit"
        n239 = property class="VI"() -> ("Front Panel.Open"=w482:bool)  [unwired: 2 in, 2 out]
        n240 = property class="App"() -> ("App.Kind"=w481:T2)  [unwired: 2 in, 2 out]
        n241 = control-ref of="Current VI Reference"() -> (w475:refnum<vi>)
        n242 = Not(x=w482) -> (.not. x?=w479:bool)
        n243 = Equal?(x=w481, y=T2."Run Time System" ("Application:Kind")) -> (x = y?=w478:bool)
        n244 = Or(x=w479, y=w478) -> (x .or. y?=w476:bool)
        n245 = Bundle By Name(cluster=w477, "Core.Current VI Reference"=w475, "Core.Close Panel on Exit?"=w476) -> (w484:T4)
        n246 = call <vilib>:"Add State(s) to Queue__jki_lib_state_machine.vi"("State(s) in (\"\")"=w486) -> ("States Out"=w485:string)  [unwired: 14 in]
      }
      frame "Error Handler" {
        # "Unhandled Error -- Display it"
        # "Handle any errors here.\nYou can also output any states to clean-up after errors occur"
        # "Clear error"
        n247 = call <vilib>:"General Error Handler.vi"("error in (no error)"=w488) -> ()  [unwired: 10 in, 5 out]
        n248 = call <vilib>:"Add State(s) to Queue__jki_lib_state_machine.vi"("State(s) in Front (\"\")"="/* Post Error States", "State(s) in (\"\")"=w492) -> ("States Out"=w491:string)  [unwired: 13 in]
      }
      frame "Exit" {
        n249 = call <vilib>:"Add State(s) to Queue__jki_lib_state_machine.vi"("State(s) in (\"\")"=w497) -> ("States Out"=w496:string)  [unwired: 14 in]
      }
      frame "---------- Data ----------" {
        # "Do not put any code in this frame.\n(It is a separator no-op. You can make a copy of this frame to create a new Data frame)"
        n250 = call <vilib>:"Add State(s) to Queue__jki_lib_state_machine.vi"("State(s) in (\"\")"=w501) -> ("States Out"=w500:string)  [unwired: 14 in]
      }
      frame "Data: Initialize" {
        (unwired) enum32{"小量程", "大量程"}."小量程" ("加计大小量程")
        w502 = FALSE  # 定时控制
        w503 = i64 0  # 起始时间
        w504 = i64 0  # 秒计数
        w506 = u16 255  # 备份控制指令
        w507 = u16 255  # 主份控制指令
        w509 = T5 {" 数据帧名称"="", " 数据"="", "备用操作符"=TRUE, "起始地址"=0, "读写标志"=0, "长度"=0}  # 信息帧
        w510 = T6 {"Current VI Reference"=refnum, "Close Panel on Exit?"=FALSE}  # Core
        n251 = Bundle("Core"=w510, "传递队列输入"=w508, "信息帧"=w509, "主份控制指令"=w507, "备份控制指令"=w506, "notifier"=w505, "秒计数"=w504, "起始时间"=w503, "定时控制"=w502) -> (w512:T4)  [unwired: 1 in]
        n252 = call <vilib>:"Add State(s) to Queue__jki_lib_state_machine.vi"("State(s) in (\"\")"=w514) -> ("States Out"=w513:string)  [unwired: 14 in]
      }
      frame "Data: Cleanup" {
        # "Cleanup any data and references, here.\n(this is called automatically, by the Macro: Exit)"
        n253 = Unbundle By Name(w515) -> ("Core.Current VI Reference"=w518:refnum<vi>)
        n254 = Close Reference(reference=w518, error in (no error)=w517) -> (error out=w516:errorcluster)
        n255 = call <vilib>:"Add State(s) to Queue__jki_lib_state_machine.vi"("State(s) in (\"\")"=w520) -> ("States Out"=w519:string)  [unwired: 14 in]
      }
      frame "---------- UI ----------" {
        # "Do not put any code in this frame.\n(It is a separator no-op. You can make a copy of this frame to create a new UI frame)"
        n256 = call <vilib>:"Add State(s) to Queue__jki_lib_state_machine.vi"("State(s) in (\"\")"=w524) -> ("States Out"=w523:string)  [unwired: 14 in]
      }
      frame "UI: Initialize" {
        # "Initialize the User Interface, here.\n(this is called automatically, by the Macro: Init)"
        n257 = property on="主份周期设置" class="RadioBtnsControl (严格)"("Value"=enum32{"160ms", "自定义", "480ms", "10ms"}."160ms" ("主份周期设置")) -> ()  [unwired: 2 in, 2 out]
        n258 = property on="备份周期设置" class="RadioBtnsControl (严格)"("Value"=enum32{"160ms", "自定义", "480ms", "10ms"}."160ms" ("主份周期设置")) -> ()  [unwired: 2 in, 2 out]
        n259 = call <vilib>:"Add State(s) to Queue__jki_lib_state_machine.vi"("State(s) in (\"\")"=w530) -> ("States Out"=w529:string)  [unwired: 14 in]
      }
      frame "UI: Cursor Set" {
        # "Argument"
        # "Set and Unset Cursor Busy.\n(Usage: \"UI: Cursor Set >> Busy|Idle\")"
        n260 = case shown="\"Idle\", 默认" w531 {
          tunnel: w533 -> [w538 w540]
          tunnel: [w537 w539] -> w532
          frame "Idle", Default {
            n261 = call <vilib>:"Unset Busy.vi"("error in (no error)"=w538) -> ("error out"=w537:errorcluster)  [unwired: 10 in]
          }
          frame "Busy" {
            n262 = call <vilib>:"Set Busy.vi"("error in (no error)"=w540) -> ("error out"=w539:errorcluster)  [unwired: 9 in, 1 out]
          }
        }
        n263 = call <vilib>:"Add State(s) to Queue__jki_lib_state_machine.vi"("State(s) in (\"\")"=w536) -> ("States Out"=w535:string)  [unwired: 14 in]
      }
      frame "UI: Front Panel State" {
        # "Set Front Panel Open or Closed\n(Usage: \"UI: Front Panel State >> Open|Close\")"
        n264 = disable-structure shown="启用" {
          disable-tunnel: w544 -> [w551 w574]
          disable-tunnel: [w550 w574] -> w543
          disable-tunnel: w542 -> [w549 _]
          disable-tunnel: w541 -> [w547 _]
          frame Disabled {
            # "Argument"
            n265 = Unbundle By Name(w549) -> ("Core.Current VI Reference"=w548:refnum<vi>)
            n266 = case shown="\"Open\", 默认" w547 {
              tunnel: w551 -> [w555 w568]
              tunnel: [w557 w569] -> w550
              tunnel: w548 -> [w556 w566]
              frame "Open", Default {
                n267 = property class="VI"(reference=w556, error in=w555) -> (reference out=w553:refnum<vi>, error out=w554:errorcluster, "Front Panel.Open"=w552:bool)
                n268 = case shown="假" w552 {
                  tunnel: [w560 w563] -> w557
                  tunnel: w554 -> [w559 w563]
                  tunnel: w553 -> [w558 _]
                  frame False {
                    n269 = invoke class="VI" method="FP.Open"(reference=w558, error in=w559, "Activate"=TRUE, "State"=T3."Standard") -> (error out=w560:errorcluster)  [unwired: 1 in, 4 out]
                  }
                  frame True {
                  }
                }
              }
              frame "Close" {
                n270 = property class="VI"(reference=w566, error in=w568) -> (reference out=w565:refnum<vi>, error out=w567:errorcluster, "Front Panel.Open"=w564:bool)
                n271 = case shown="真" w564 {
                  tunnel: [w570 w573] -> w569
                  tunnel: w567 -> [w570 w572]
                  tunnel: w565 -> [_ w571]
                  frame False {
                  }
                  frame True {
                    n272 = invoke class="VI" method="FP.Close"(reference=w571, error in=w572) -> (error out=w573:errorcluster)  [unwired: 1 in, 2 out]
                  }
                }
              }
            }
          }
          frame Enabled {
          }
        }
        n273 = call <vilib>:"Add State(s) to Queue__jki_lib_state_machine.vi"("State(s) in (\"\")"=w546) -> ("States Out"=w545:string)  [unwired: 14 in]
      }
      frame "---------- Macro ----------" {
        # "Do not put any code in this frame.\n(It is a separator no-op. You can make a copy of this frame to create a new Macro frame)"
        n274 = call <vilib>:"Add State(s) to Queue__jki_lib_state_machine.vi"("State(s) in (\"\")"=w578) -> ("States Out"=w577:string)  [unwired: 14 in]
      }
      frame "Macro: Initialize" {
        w579 = "Data: Initialize\nInitialize Core Data\nUI: Initialize\nUI: Front Panel State >> Open"  # Data: Initialize Initialize Core Data UI: Initialize UI: Front Panel State >> Open
        # "Initialization Macro\n(This is called once, when the VI starts)"
        n275 = call <vilib>:"Add State(s) to Queue__jki_lib_state_machine.vi"("State(s) in Front (\"\")"=w579, "State(s) in (\"\")"=w583) -> ("States Out"=w582:string)  [unwired: 13 in]
      }
      frame "Macro: Exit" {
        # "Exit Macro\n(This is called once, when the VI exits)"
        n276 = Unbundle By Name(w590) -> ("Core.Close Panel on Exit?"=w589:bool)
        n277 = Select(t="UI: Front Panel State >> Close", s=w589, f="") -> (s? t:f=w586:string)
        n278 = call <vilib>:"Add State(s) to Queue__jki_lib_state_machine.vi"("State(s) in (\"\")"=w586, "State(s) at Back (\"\")"="Data: Cleanup\nExit") -> ("States Out"=w584:string)  [unwired: 13 in]
        n279 = call <vilib>:"Add State(s) to Queue__jki_lib_state_machine.vi"("State(s) in Front (\"\")"=w584, "State(s) in (\"\")"=w593) -> ("States Out"=w592:string)  [unwired: 13 in]
      }
      frame "----------Request----------" {
        # "Template Separator\n(You can make a copy of, or modify, this frame)"
        n280 = call <vilib>:"Add State(s) to Queue__jki_lib_state_machine.vi"("State(s) in (\"\")"=w597) -> ("States Out"=w596:string)  [unwired: 14 in]
      }
      frame "Request:Write" {
        n281 = in-place {
          in-place-border: w601 -> [w608]
          in-place-border: [w607] -> w600
          in-place-border: w598 -> [w606]
          n282 = in-place-cluster #18(w602) -> ("传递队列输入"=w612:refnum<queue>, "信息帧"=w611:T5)  [unwired: 1 out]
          n283 = in-place {
            in-place-border: w606 -> [w613]
            n284 = in-place-cluster #19(w611) -> ("数据"=w618:string)  [unwired: 5 out]
            n285 = in-place-cluster #19("数据帧名称"=w613, "数据"=w618, "备用操作符"=TRUE, "起始地址"=0, "读写标志"=1, "长度"=0) -> (w610:T5)
          }
          n286 = Enqueue Element(queue=w612, element=w610, error in (no error)=w608) -> (queue out=w609:refnum<queue>, error out=w607:errorcluster)  [unwired: 1 in, 1 out]
          n287 = in-place-cluster #18("传递队列输入"=w609, "信息帧"=w610, "主份控制指令"=u16 255) -> (w599:T4)
        }
        n288 = call <vilib>:"Add State(s) to Queue__jki_lib_state_machine.vi"("State(s) in (\"\")"=w604) -> ("States Out"=w603:string)  [unwired: 14 in]
      }
      frame "Config:Write" {
        n289 = in-place {
          in-place-border: w622 -> [w628]
          in-place-border: [w627] -> w621
          in-place-border: w619 -> [w626]
          n290 = in-place-cluster #20(w623) -> ("传递队列输入"=w632:refnum<queue>, "信息帧"=w631:T5)
          n291 = in-place {
            in-place-border: w626 -> [w633]
            n292 = in-place-cluster #21(w631) -> ("数据"=w638:string)  [unwired: 5 out]
            n293 = in-place-cluster #21("数据帧名称"=w633, "数据"=w638, "备用操作符"=TRUE, "起始地址"=0, "读写标志"=2, "长度"=0) -> (w630:T5)
          }
          n294 = Enqueue Element(queue=w632, element=w630, error in (no error)=w628) -> (queue out=w629:refnum<queue>, error out=w627:errorcluster)  [unwired: 1 in, 1 out]
          n295 = in-place-cluster #20("传递队列输入"=w629, "信息帧"=w630) -> (w620:T4)
        }
        n296 = call <vilib>:"Add State(s) to Queue__jki_lib_state_machine.vi"("State(s) in (\"\")"=w625) -> ("States Out"=w624:string)  [unwired: 14 in]
      }
      frame "Request:OPEN1553B" {
        n297 = in-place {
          in-place-border: w642 -> [w649]
          in-place-border: [w648] -> w641
          in-place-border: w639 -> [w646]
          n298 = in-place-cluster #22(w643) -> ("传递队列输入"=w652:refnum<queue>, "信息帧"=w647:T5)
          n299 = in-place {
            in-place-border: w646 -> [w653]
            n300 = in-place-cluster #23(w647) -> ()  [unwired: 6 out]
            n301 = in-place-cluster #23("数据帧名称"=w653, "数据"="$B\n", "备用操作符"=TRUE, "起始地址"=0, "读写标志"=1, "长度"=0) -> (w651:T5)
          }
          n302 = Enqueue Element(queue=w652, element=w651, error in (no error)=w649) -> (queue out=w650:refnum<queue>, error out=w648:errorcluster)  [unwired: 1 in, 1 out]
          n303 = in-place-cluster #22("传递队列输入"=w650, "信息帧"=w647) -> (w640:T4)
        }
        n304 = call <vilib>:"Add State(s) to Queue__jki_lib_state_machine.vi"("State(s) in (\"\")"=w645) -> ("States Out"=w644:string)  [unwired: 14 in]
      }
      frame "Request:Close1553B" {
        n305 = in-place {
          in-place-border: w661 -> [w670]
          in-place-border: [w669] -> w660
          n306 = in-place-cluster #24(w662) -> ("传递队列输入"=w672:refnum<queue>, "信息帧"=w666:T5)
          n307 = in-place {
            n308 = in-place-cluster #25(w666) -> ()  [unwired: 6 out]
            n309 = in-place-cluster #25("数据帧名称"="1553B_CMD", "数据"="$", "备用操作符"=TRUE, "起始地址"=0, "读写标志"=1, "长度"=0) -> (w671:T5)
          }
          n310 = in-place {
            n311 = in-place-cluster #26(w666) -> ()  [unwired: 6 out]
            n312 = in-place-cluster #26("数据帧名称"="1553B_CMD", "数据"="$Z\n", "备用操作符"=TRUE, "起始地址"=0, "读写标志"=1, "长度"=0) -> (w667:T5)
          }
          n313 = Enqueue Element(queue=w672, element=w671, error in (no error)=w670) -> (queue out=w668:refnum<queue>, error out=w669:errorcluster)  [unwired: 1 in, 1 out]
          n314 = Enqueue Element(queue=w668, element=w667) -> (queue out=w665:refnum<queue>)  [unwired: 2 in, 2 out]
          n315 = in-place-cluster #24("传递队列输入"=w665, "信息帧"=w666) -> (w659:T4)
        }
        n316 = call <vilib>:"Add State(s) to Queue__jki_lib_state_machine.vi"("State(s) in (\"\")"=w664) -> ("States Out"=w663:string)  [unwired: 14 in]
      }
      frame "Request:Read" {
        n317 = in-place {
          in-place-border: w687 -> [w692]
          in-place-border: [w691] -> w686
          n318 = in-place-cluster #27(w688) -> ("传递队列输入"=w696:refnum<queue>, "信息帧"=w695:T5)
          n319 = in-place {
            n320 = in-place-cluster #28(w695) -> ("数据"=w701:string)  [unwired: 5 out]
            n321 = in-place-cluster #28("数据帧名称"="GNSS1", "数据"=w701, "备用操作符"=TRUE, "起始地址"=0, "读写标志"=0, "长度"=0) -> (w694:T5)
          }
          n322 = Enqueue Element(queue=w696, element=w694, error in (no error)=w692) -> (queue out=w693:refnum<queue>, error out=w691:errorcluster)  [unwired: 1 in, 1 out]
          n323 = in-place-cluster #27("传递队列输入"=w693, "信息帧"=w694) -> (w685:T4)
        }
        n324 = call <vilib>:"Add State(s) to Queue__jki_lib_state_machine.vi"("State(s) in (\"\")"=w690) -> ("States Out"=w689:string)  [unwired: 14 in]
      }
      frame "----------Usr----------" {
        # "Template Separator\n(You can make a copy of, or modify, this frame)"
        n325 = call <vilib>:"Add State(s) to Queue__jki_lib_state_machine.vi"("State(s) in (\"\")"=w706) -> ("States Out"=w705:string)  [unwired: 14 in]
      }
      frame "Exit:all" {
        n326 = call <vilib>:"Add State(s) to Queue__jki_lib_state_machine.vi"("State(s) in Front (\"\")"="Macro: Exit", "State(s) in (\"\")"=w711) -> ("States Out"=w710:string)  [unwired: 13 in]
      }
    }
  }
  n327 = while {
    tunnel: "notifier" -> [w802]
    stop <- w801 stop-if-true
    n328 = call "stop_message.vi"("notifier"=w802) -> ("Exit？"=w801:bool)  [unwired: 9 in, 1 out]
    n329 = Wait Until Next ms Multiple(millisecond multiple=u32 200 ("毫秒倍数")) -> ()  [unwired: 1 out]
    n330 = call <vilib>:"Read.vi"("Register name"="AIs") -> ("Register value"=w799:variant)  [unwired: 11 in, 3 out]
    n331 = call-poly <vilib>:"Convert.vi"("Register value in"=w799) -> ("Register value out"=w798:sgl[])  [unwired: 13 in, 1 out]
    n332 = for {
      N: 9 -> [_]
      tunnel: w798 -> [w810] mode=indexing
      shift-right: [w811] -> w796
      shift-left: "模拟量\n\n" -> [w804]
      tunnel: string[] ["外部模拟量", "A_LTU电源遥测", "B_LTU电源遥测", "G1陀螺电源遥测", "G2陀螺电源遥测", "G3陀螺电源遥测", "A1加计电源遥测", "A2加计电源遥测", "A3加计电源遥测"] -> [w805] mode=indexing
      n333 = Concatenate Strings(w805, "                     " ("字符串")) -> (w808:string)
      n334 = String Subset(string=w808, length (rest)=16 ("长度（剩余）")) -> (substring=w806:string)  [unwired: 1 in]
      n335 = Number To Fractional String(number=w810, width (-)=i16 6 ("宽度(-)"), precision (6)=i16 3 ("精度(6)")) -> (F-format string=w813:string)  [unwired: 1 in]
      n336 = Concatenate Strings(w804, w806, w813, "\n") -> (w811:string)
    }
    "模拟量显示区" <- w796
    n337 = call <vilib>:"Read.vi"("Register name"="1553BZhuFenRecv_stat" ("字符串")) -> ("Register value"=w792:variant)  [unwired: 11 in, 3 out]
    n338 = call <vilib>:"Read.vi"("Register name"="1553BBeiFenRecv_stat" ("字符串")) -> ("Register value"=w738:variant)  [unwired: 11 in, 3 out]
    n339 = Variant To Data(type=T7 {"G1陀螺脉冲数"=0, "G2陀螺脉冲数"=0, "G3陀螺脉冲数"=0, "A1加速度计脉冲数"=0, "A2加速度计脉冲数"=0, "A3加速度计脉冲数"=0, "G1陀螺自检状态"=0, "G1陀螺光路温度"=0, "G2陀螺自检状态"=0, "G2陀螺光路温度"=0, "G3陀螺自检状态"=0, "G3陀螺光路温度"=0, "A1自检状态"=0, "A1幅值"=0, "A2自检状态"=0, "A2幅值"=0, "A3自检状态"=0, "A3幅值"=0, "IF1电路温度"=0, "IF2电路温度"=0, "IF3电路温度"=0, "温控自检字"=0, "加计温度1"=0, "加计温度2"=0, "LTU状态"=0, "帧计数"=0, "G1陀螺光路温度E-2"=0, "G2陀螺光路温度E-2"=0, "G3陀螺光路温度E-2"=0, "G1陀螺电路温度E-2"=0, "G2陀螺电路温度E-2"=0, "G3陀螺电路温度E-2"=0} ("输入簇"), Variant=w792) -> (data=w791:T7)  [unwired: 1 in, 1 out]
    n340 = Variant To Data(type=T7 {"G1陀螺脉冲数"=0, "G2陀螺脉冲数"=0, "G3陀螺脉冲数"=0, "A1加速度计脉冲数"=0, "A2加速度计脉冲数"=0, "A3加速度计脉冲数"=0, "G1陀螺自检状态"=0, "G1陀螺光路温度"=0, "G2陀螺自检状态"=0, "G2陀螺光路温度"=0, "G3陀螺自检状态"=0, "G3陀螺光路温度"=0, "A1自检状态"=0, "A1幅值"=0, "A2自检状态"=0, "A2幅值"=0, "A3自检状态"=0, "A3幅值"=0, "IF1电路温度"=0, "IF2电路温度"=0, "IF3电路温度"=0, "温控自检字"=0, "加计温度1"=0, "加计温度2"=0, "LTU状态"=0, "帧计数"=0, "G1陀螺光路温度E-2"=0, "G2陀螺光路温度E-2"=0, "G3陀螺光路温度E-2"=0, "G1陀螺电路温度E-2"=0, "G2陀螺电路温度E-2"=0, "G3陀螺电路温度E-2"=0} ("输入簇"), Variant=w738) -> (data=w739:T7)  [unwired: 1 in, 1 out]
    n341 = Unbundle By Name(w791) -> ("G1陀螺自检状态"=w780:u8, "G2陀螺自检状态"=w773:u8, "G3陀螺自检状态"=w772:u8, "A1自检状态"=w771:u8, "A2自检状态"=w770:u8, "A3自检状态"=w769:u8, "温控自检字"=w790:u8, "LTU状态"=w789:u8)  [unwired: 1 out]
    n342 = Unbundle By Name(w739) -> ("G1陀螺自检状态"=w744:u8, "G2陀螺自检状态"=w751:u8, "G3陀螺自检状态"=w752:u8, "A1自检状态"=w753:u8, "A2自检状态"=w754:u8, "A3自检状态"=w755:u8, "温控自检字"=w740:u8, "LTU状态"=w741:u8)  [unwired: 1 out]
    n343 = Number To Boolean Array(number=w770) -> (Boolean array=w727:bool[])
    n344 = Number To Boolean Array(number=w769) -> (Boolean array=w726:bool[])
    n345 = Number To Boolean Array(number=w754) -> (Boolean array=w722:bool[])
    n346 = Number To Boolean Array(number=w755) -> (Boolean array=w721:bool[])
    n347 = Number To Boolean Array(number=w790) -> (Boolean array=w725:bool[])
    n348 = Number To Boolean Array(number=w789) -> ()  [unwired: 1 out]
    n349 = Number To Boolean Array(number=w740) -> (Boolean array=w720:bool[])
    n350 = Number To Boolean Array(number=w741) -> ()  [unwired: 1 out]
    n351 = Number To Boolean Array(number=w753) -> (Boolean array=w723:bool[])
    n352 = Number To Boolean Array(number=w771) -> (Boolean array=w728:bool[])
    n353 = Number To Boolean Array(number=w772) -> (Boolean array=w729:bool[])
    n354 = Number To Boolean Array(number=w752) -> (Boolean array=w724:bool[])
    n355 = Number To Boolean Array(number=w780) -> (Boolean array=w788:bool[])
    n356 = Number To Boolean Array(number=w744) -> (Boolean array=w742:bool[])
    n357 = Number To Boolean Array(number=w773) -> (Boolean array=w786:bool[])
    n358 = Number To Boolean Array(number=w751) -> (Boolean array=w743:bool[])
    n359 = Index Array(array=w729) -> (element #3=→"主份G3加电状态":bool)  [unwired: 3 in, 2 out]
    n360 = Index Array(array=w726) -> (element #3=→"主份A3加电状态":bool)  [unwired: 3 in, 2 out]
    n361 = Index Array(array=w725, index #1=6 ("索引")) -> (element #1=→"主份温控工作状态":bool, element #2=→"主份温控健康状态":bool)  [unwired: 1 in]
    n362 = Index Array(array=w724) -> (element #3=→"备份G3加电状态":bool)  [unwired: 3 in, 2 out]
    n363 = Index Array(array=w721) -> (element #3=→"备份A3加电状态":bool)  [unwired: 3 in, 2 out]
    n364 = Index Array(array=w720, index #1=6 ("索引")) -> (element #1=→"备份温控工作状态":bool, element #2=→"备份温控健康状态":bool)  [unwired: 1 in]
    n365 = Index Array(array=w788) -> (element #3=→"主份G1加电状态":bool)  [unwired: 3 in, 2 out]
    n366 = Index Array(array=w786) -> (element #3=→"主份G2加电状态":bool)  [unwired: 3 in, 2 out]
    n367 = Index Array(array=w728) -> (element #3=→"主份A1加电状态":bool)  [unwired: 3 in, 2 out]
    n368 = Index Array(array=w727) -> (element #3=→"主份A2加电状态":bool)  [unwired: 3 in, 2 out]
    n369 = Index Array(array=w742) -> (element #3=→"备份G1加电状态":bool)  [unwired: 3 in, 2 out]
    n370 = Index Array(array=w743) -> (element #3=→"备份G2加电状态":bool)  [unwired: 3 in, 2 out]
    n371 = Index Array(array=w723) -> (element #3=→"备份A1加电状态":bool)  [unwired: 3 in, 2 out]
    n372 = Index Array(array=w722) -> (element #3=→"备份A2加电状态":bool)  [unwired: 3 in, 2 out]
    n373 = call "陀螺状态自检.vi"("G123"="G1", "陀螺自检状态字"=w780) -> ("连接的字符串"=w768:string)  [unwired: 9 in]
    n374 = call "陀螺状态自检.vi"("G123"="G2", "陀螺自检状态字"=w773) -> ("连接的字符串"=w767:string)  [unwired: 9 in]
    n375 = call "陀螺状态自检.vi"("G123"="G3", "陀螺自检状态字"=w772) -> ("连接的字符串"=w766:string)  [unwired: 9 in]
    n376 = call "陀螺状态自检.vi"("G123"="G1", "陀螺自检状态字"=w744) -> ("连接的字符串"=w756:string)  [unwired: 9 in]
    n377 = call "陀螺状态自检.vi"("G123"="G2", "陀螺自检状态字"=w751) -> ("连接的字符串"=w757:string)  [unwired: 9 in]
    n378 = call "陀螺状态自检.vi"("G123"="G3", "陀螺自检状态字"=w752) -> ("连接的字符串"=w758:string)  [unwired: 9 in]
    n379 = call "加计状态自检.vi"("G123"="A1", "加速度计自检状态字"=w771) -> ("连接的字符串"=w765:string)  [unwired: 9 in]
    n380 = call "加计状态自检.vi"("G123"="A2", "加速度计自检状态字"=w770) -> ("连接的字符串"=w764:string)  [unwired: 9 in]
    n381 = call "加计状态自检.vi"("G123"="A3", "加速度计自检状态字"=w769) -> ("连接的字符串"=w763:string)  [unwired: 9 in]
    n382 = call "加计状态自检.vi"("G123"="A1", "加速度计自检状态字"=w753) -> ("连接的字符串"=w759:string)  [unwired: 9 in]
    n383 = call "加计状态自检.vi"("G123"="A2", "加速度计自检状态字"=w754) -> ("连接的字符串"=w760:string)  [unwired: 9 in]
    n384 = call "加计状态自检.vi"("G123"="A3", "加速度计自检状态字"=w755) -> ("连接的字符串"=w761:string)  [unwired: 9 in]
    n385 = Concatenate Strings(w768, w767, w766, w765, w764, w763) -> (→"主份自检状态及船舱标志":string)
    n386 = Concatenate Strings(w756, w757, w758, w759, w760, w761) -> (→"备份自检状态及船舱标志":string)
  }
